vi "SSA_Template.vi"(0 "Reac Info":string[][](array[string])=[["Degradation_GFP", "", "false", "false", "Cell", "1", "GFP", "1.0", "true", "0", "", "", "0", "", "1", "kd", "0.0075"], ["Degradation_TetR", "", "false", "false", "Cell", "1", "TetR", "1.0", "true", "0", "", "", "0", "", "1", "kd", "0.0075"], ["Degradation_LacI", "", "false", "false", "Cell", "1", "LacI", "1.0", "true", "0", "", "", "0", "", "1", "kd", "0.0075"], ["R_abstracted_production_P1", "", "false", "false", "Cell", "0", "", "", "true", "1", "GFP", "10.0", "1", "LacI", "6", "RNAP, ng__P1, Ko__P1, ko__P1, nc__LacI_P1, Kr__LacI_P1", "30.0, 2.0, 0.033, 0.05, 2.0, 0.5"], ["R_abstracted_production_P2", "", "false", "false", "Cell", "0", "", "", "true", "1", "GFP", "10.0", "1", "TetR", "6", "RNAP, ng__P2, Ko__P2, ko__P2, nc__TetR_P2, Kr__TetR_P2", "30.0, 2.0, 0.033, 0.05, 2.0, 0.5"]], 1 "Ex_Mod_IDs":string[](array[string])=["LacI", "TetR"], 2 "Idx of Mod in Sp IDs":i32[](array[numeric])=[1, 4], 5 "Math Expressions":string[](array[string])=["kd*GFP", "kd*TetR", "kd*LacI", "ko__P1*ng__P1*Ko__P1*RNAP/(1+Ko__P1*RNAP+(Kr__LacI_P1*LacI)^nc__LacI_P1)", "ko__P2*ng__P2*Ko__P2*RNAP/(1+Ko__P2*RNAP+(Kr__TetR_P2*TetR)^nc__TetR_P2)"], 7 "Species Info":string[][](array[string])=[["GFP", "", "Cell", "0.0", "NaN", "", "true", "false", "false", "null"], ["LacI", "", "Cell", "0.0", "NaN", "", "true", "true", "false", "null"], ["P1", "", "Cell", "2.0", "NaN", "", "true", "false", "false", "null"], ["P2", "", "Cell", "2.0", "NaN", "", "true", "false", "false", "null"], ["TetR", "", "Cell", "0.0", "NaN", "", "true", "true", "false", "null"]], 9 "Parameter info":string[][](array[string])=[["ko_r", "Reverse RNAP binding rate", "1.0", "", "true"], ["nr", "Initial RNAP count", "30.0", "", "true"], ["np", "Stoichiometry of production", "10.0", "", "true"], ["kr_r", "Reverse repression binding rate", "1.0", "", "true"], ["ka_f", "Forward activation binding rate", "0.0033", "", "true"], ["kecdiff", "Extracellular diffusion rate", "1.0", "", "true"], ["ko", "Open complex production rate", "0.05", "", "true"], ["kmdiff_f", "Forward membrane diffusion rate", "1.0", "", "true"], ["kecd", "Extracellular degradation rate", "0.005", "", "true"], ["kc_r", "Reverse complex formation rate", "1.0", "", "true"], ["kr_f", "Forward repression binding rate", "0.5", "", "true"], ["ka_r", "Reverse activation binding rate", "1.0", "", "true"], ["nc", "Stoichiometry of binding", "2.0", "", "true"], ["kao_r", "Reverse activated RNAP binding rate", "1.0", "", "true"], ["kd", "Degradation rate", "0.0075", "", "true"], ["kb", "Basal production rate", "1.0E-4", "", "true"], ["ng", "Initial promoter count", "2.0", "", "true"], ["ka", "Activated production rate", "0.25", "", "true"], ["kao_f", "Forward activated RNAP binding rate", "1.0", "", "true"], ["kmdiff_r", "Reverse membrane diffusion rate", "0.01", "", "true"], ["ko_f", "Forward RNAP binding rate", "0.033", "", "true"], ["kc_f", "Forward complex formation rate", "0.05", "", "true"], ["High", "", "120.0", "", "true"], ["HighTime", "", "1000.0", "", "true"], ["HighTime2", "", "2000.0", "", "true"]], 11 "Local Parameter Info":string[][](array[string])=[["kd", "0.0075"], ["kd", "0.0075"], ["kd", "0.0075"], ["RNAP", "30.0"], ["ng__P1", "2.0"], ["Ko__P1", "0.033"], ["ko__P1", "0.05"], ["nc__LacI_P1", "2.0"], ["Kr__LacI_P1", "0.5"], ["RNAP", "30.0"], ["ng__P2", "2.0"], ["Ko__P2", "0.033"], ["ko__P2", "0.05"], ["nc__TetR_P2", "2.0"], ["Kr__TetR_P2", "0.5"]]) -> ()   [LabVIEW 2014]
uses:
  <vilib>/Analysis/Matrix/Datatypes/RealMatrix.ctl
  Modifier Control.ctl
  Event Info.ctl
  <vilib>/Utility/error.llb/DialogType.ctl
  ValSubsCtrl.ctl
  Trigger Status Bar.vi
  <vilib>/Utility/file.llb/Write To Spreadsheet File (DBL).vi
  <vilib>/Utility/file.llb/Write To Spreadsheet File (string).vi
  <vilib>/Analysis/Matrix/Numeric/Conversions/Matrix To Array - RM.vi
  <vilib>/regexp/Match Regular Expression.xnode
  <vilib>/Analysis/Matrix/NI_Matrix.lvlib
  <vilib>/gmath/NI_Gmath.lvlib
  <vilib>/Utility/file.llb/Read From Spreadsheet File (DBL).vi
panel:
  out "Reaction Math":string[][](array[string])
  out "Trig  MSW":bool=TRUE
  out "Plot colors":u32[](array[numeric])
  out "Plot Names":string[](array[string])
  out "Sp_Init_Amnt":string[](array[string])
  out "Trig Ext Mod Selection":bool=TRUE
  out "FuncCnt":i32
  out "Functions":string[][](array[string])
  out "Fn Arg Cnt":string[](array[string])
  out "Priority":dbl[](array[numeric])
  out "Delay Val Tot":dbl[](array[numeric])
  out "Flag":i32[](array[numeric])
  out "Delay":dbl[](array[numeric])
  out "Delay Val":dbl
  out "Event Idx":i32
  out "All Variables":string[](array[string])
  out "Time Limit":dbl
  out "ModTimeSym":string
  out "CompSize":string[](array[string])
  out "CompID":string[](array[string])
  out "Comp Def":string[][](array[string])
  out "Rules":string[][](array[string])
  out "RulesCnt":i32
  in  "Run":bool
  in  "stop":bool
  in  "Stop Main":bool
  out "Sp_Name":string[](array[string])
  out "Reac IDx":i32
  out "T=inf":bool
  out "Nxt Sp State (N)":dbl[](array[numeric])
  out "Propensities":dbl[](array[numeric])
  out "tau":dbl
  out "T":dbl[](array[numeric])
  out "Nxt T":dbl
  out "AppPath":string
  out "path":path
  in  "Shut Down":bool
  out "Default Stoich":dbl[](array[numeric])
  in  "Event Info":T1
  in  "Model Name 2":string="nand_RB"
  in  "Model Name":string="nand_RB"
  out "Reactant Matrix":T2
  out "Sp Ids":string[](array[string])
  out "Delta Matrix":T2
  out "XY Graph":cluster{"T":dbl[], dbl[]}[](graph)
  in  "Include Cello UCF":bool
  in  "Set Time Limit":string="100"
  in  "Continous Simulation":bool
  in  "Simulate SBML Events":bool
  in  "Threshold Value Analysis":bool
  in  "Modifier Degradation":bool
  in  "Slider":bool
  out "Assign Val":string[][](array[string])
  out "Var Idx":i32[](array[numeric])
  out "output array":T2
  out "RulVarIdx":i32[](array[numeric])
  out "DelMatRul":T2
  out "Init Sp State (S)":string[](array[string])
  out "DelMatOrigSize":i32
  out "Assign Var Idx":i32[][](array[numeric])
  out "Math Op":string[](array[string])
  out "Math Val":string[](array[string])
  in  "Events Info":string[][](table)=[["event0", "true", "true", "true", "t >= HighTime", "TetR = High"], ["event1", "true", "true", "true", "t >= HighTime2", "LacI = High"]]
  out "Log Data matrix":dbl[][](array[numeric]) format="%0.3f"
  out "All Param IDs":string[](array[string])
  out "All Param Vals":string[](array[string])
  out "Log Data":dbl[](array[numeric])
  out "Reac to execute":dbl[](array[numeric])
  out "Output Equations":string[](array[string])
  out "Nxt Sp State (S)":string[](array[string])
  out "All Param Names":string[](array[string])
  out "Equations":string[](array[string])
  out "Init Sp State (N)":dbl[](array[numeric])
  out "a0*r2":dbl
  out "Sum of Propensities for U":dbl
  out "Sum>a0*r2":bool
  out "r1":dbl
  out "L_cnt":i32
  out "r2":dbl
  out "a0":dbl
  out "Sp Data":dbl[][](array[numeric]) format="%0.3f"
  in  "External Modifiers":T3[](array[typedef]) {"Dial" scale=0.0..100.0 scale format="%#_3g"}
  in  "Boolean":bool=TRUE
  out "Est Thresh Val":dbl
  in  "Logic Verification":bool
  in  "Simulation Speed (ms)":u32=30
  out "DataLog":path
  out "All Param Values":string[](array[string])
  # "Virtual Laboratory Instrument for Stochastic Simulations"
  # "Settings"
  # "Yes"
  # "No"
  # "Manual"
  # "Auto"
  # "Model Parameters"
  # "Global Parameters"
  # "Local Parameters"
  # "ID"
  # "Name"
  # "Value"
  # "ID"
  # "Value"
  # "Runtime Simulation\nOptions"
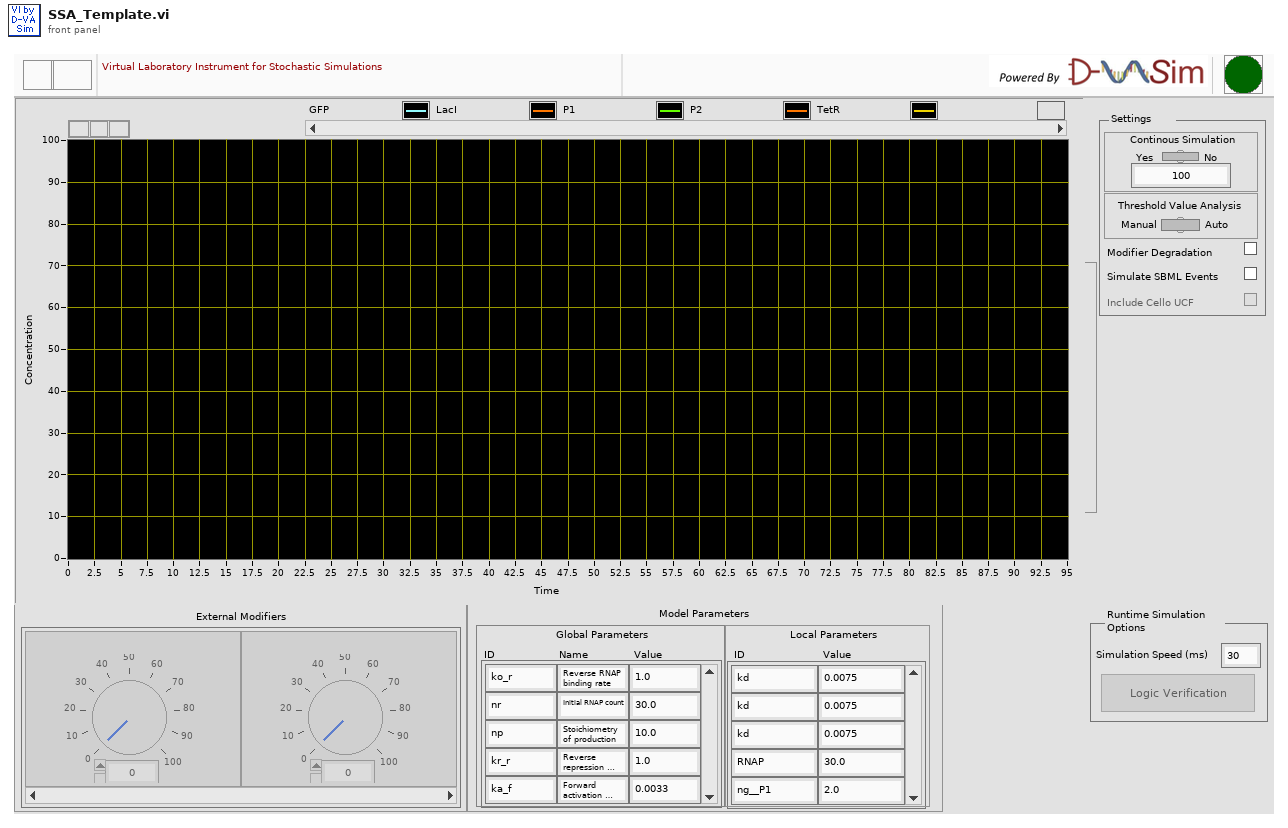
[diagram p1: front panel]
types:
  T1 = typedef "Event Info.ctl" = cluster{"Math Var":string[], "Math Op":string[], "Math Val":string[], "Assign Var":string[][], "Assign Op":string[][], "Assign Val":string[][], "Var Idx":i32[], "Assign Var Idx":i32[][], "Delay":string[], "Priority":string[]}
  T2 = typedef "NI_Matrix.lvlib/RealMatrix.ctl" = dbl[][]
  T3 = typedef "Modifier Control.ctl" = cluster{"Dial":dbl, "String 2":string}
  T4 = typedef "DialogType.ctl" = u16
  T5 = typedef "Model Information.ctl" = cluster{"ID":string, "Name":string, "Substance Units":string, "Time Units":string, "Volume Units":string, "Area Units":string, "Length Units":string, "Extent Units":string, "Conversion Factor":string, "Model Components":string}
  T6 = cluster{"Model Info":T5, "SpCnt":i32, "Species Info":string[][], "Pr_Cnt":i32, "Parameter info":string[][], "ReacCnt":i32, "Reaction Info":string[][], "Math Expressions":string[][], "EventsCnt":i32, "Event Info":string[][], "UnitsDefCnt":i32, "Units Def":string[][], "CompCnt":i32, "Comp Def":string[][], "Mod_ID":string[], "Mod_Idx":i32[], "RulesCnt":i32, "Rules":string[][], "FuncCnt":i32, "Functions":string[][], "InitAssign Cnt":i32, "Init Assigns":string[][], "ConstraintsCnt":i32, "Constraints":string[][], "Fn Arg Cnt":string[]}
  T7 = enum8{"Enabled", "Disabled", "Disabled and Grayed Out"}
  T8 = typedef "ValSubsCtrl.ctl" = cluster{"All Param Names":string[], "All Param Values":string[], "Sp IDs":string[], "Sp States":string[], "Input Equations":string[], "CompID":string[], "CompSize":string[], "T-Sym":string, "T":dbl}
  T9 = typedef "Threshold Set.ctl" = cluster{"Start at":dbl, "Increment of":dbl, "Stop at":dbl, "No. of iterations":dbl, "Assumed Time Delay":dbl, "Th high":dbl, "Verification RT":dbl, "Settling Time":i32, "Name of Output":string, "Th Low":dbl}
  T10 = enum32{"invalid app kind", "Development System", "Run Time System", "Student Edition", "Embedded LabVIEW", "Evaluation", "Custom"}
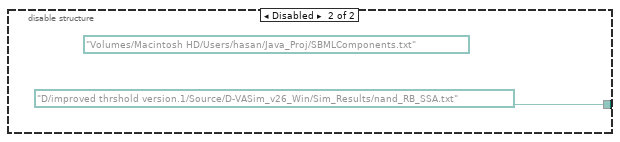
[diagram p2: hidden frame]
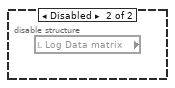
[diagram p3: hidden frame]
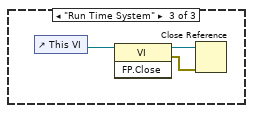
[diagram p5: hidden frame]
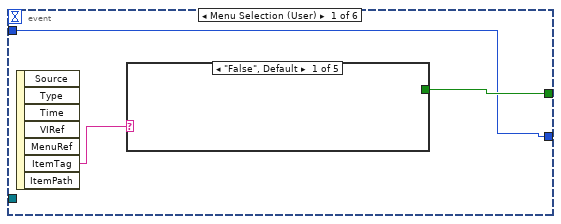
[diagram p6: hidden frame]
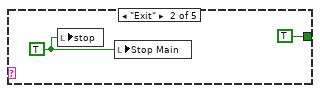
[diagram p7: hidden frame]
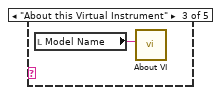
[diagram p8: hidden frame]
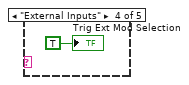
[diagram p9: hidden frame]
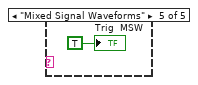
[diagram p10: hidden frame]
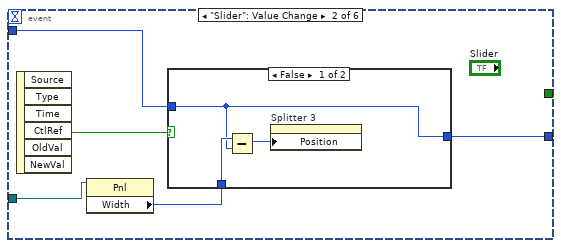
[diagram p11: hidden frame]
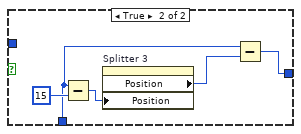
[diagram p12: hidden frame]
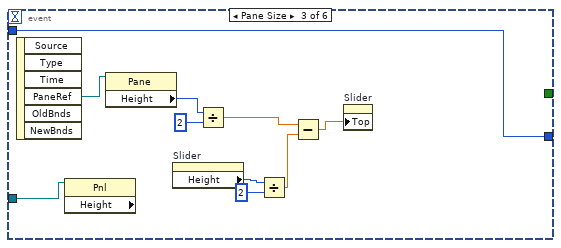
[diagram p13: hidden frame]
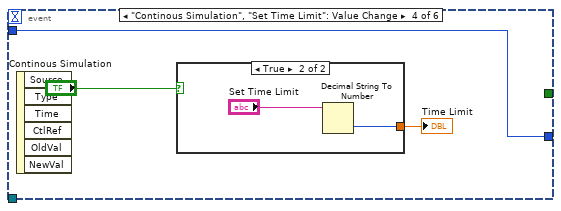
[diagram p14: hidden frame]
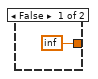
[diagram p15: hidden frame]
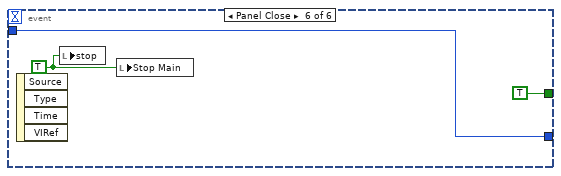
[diagram p16: hidden frame]
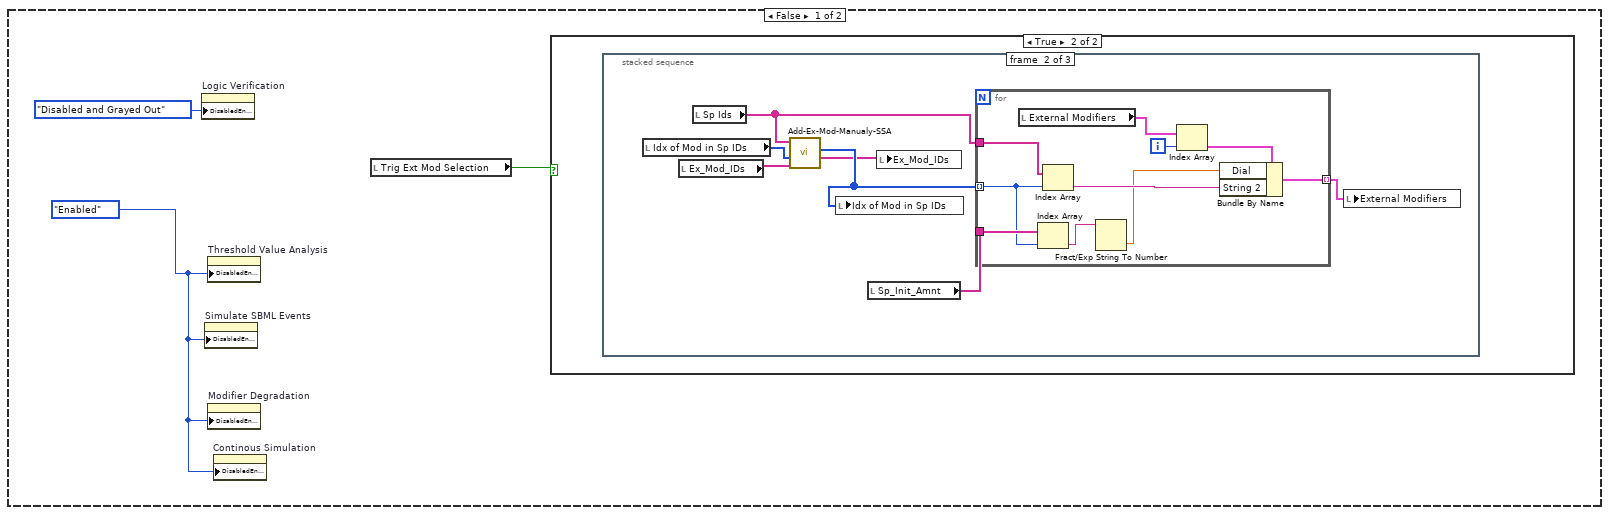
[diagram p17: hidden frame]
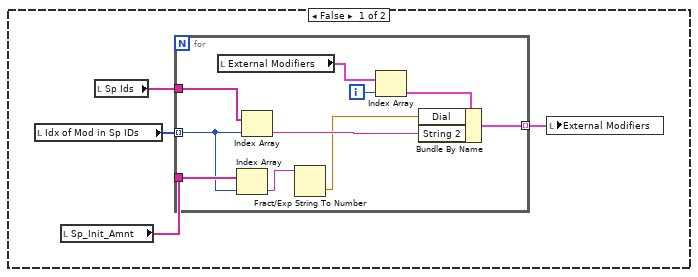
[diagram p18: hidden frame]
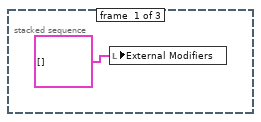
[diagram p19: hidden frame]
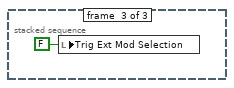
[diagram p20: hidden frame]
diagram:
  (unwired) 928 ("Splitter Position")
  w9 = T4 2 items=["no dialog", "OK message", "continue or stop message", "OK message + warnings", "continue/stop + warnings"] ("type of dialog (OK msg:1)")
  n1 = flat-sequence {
    tunnel: [w11] -> w4
    tunnel: w4 -> [w36]
    tunnel: [w69] -> w3
    frame #0 {
      n2 = Current VI's Path() -> (path=w21:path)
      n3 = Path To String(path=w21) -> (string=w20:string)
      n4 = Match Pattern(string=w20, regular expression="Sim_Results\\" ("string")) -> (before substring=w18:string)  [unwired: 1 in, 3 out]
      n5 = Concatenate Strings(w18, "Sim_Results\\" ("string")) -> (w16:string)
      "AppPath" <- w16
      n6 = disable-structure shown="Enabled" {
        disable-tunnel: [w31 path "D:/improved thrshold version.1/Source/D-VASim_v26_Win/Sim_Results/nand_RB_SSA.txt" ("SBML File")] -> w11
        disable-tunnel: w16 -> [w22 _]
        frame Enabled {
          # "Reference convert into path"
          n7 = control-ref of="This VI"() -> (w30:refnum<vi>)
          n8 = property class="VI"(reference=w30) -> ("Name"=w29:string)  [unwired: 1 in, 2 out]
          n9 = Search and Replace String(input string=w29, search string=".vi", replace string="") -> (result string=w26:string)  [unwired: 5 in, 3 out]
          n10 = Concatenate Strings(w26, ".txt" ("search string")) -> (w24:string)
          n11 = local write "Model Name"(w26) -> ()
          n12 = Concatenate Strings(w22, w24) -> (w23:string)
          n13 = String To Path(string=w23) -> (path=w31:path)
        }
        frame Disabled {
          (unwired) path "/Volumes/Macintosh HD/Users/hasan/Java_Proj/SBMLComponents.txt" ("SBML File")
        }
      }
      "path" <- w11
      n14 = property on="XY Graph" class="XYGraph (strict)"("LegScrollVis"=TRUE ("Legend:Scrollbar Visible")) -> ()  [unwired: 2 in, 2 out]
      n15 = property on="XY Graph" class="XYGraph (strict)"("LegAutosize"=FALSE ("Legend:Autosize"), "Plot.Plot Name"="") -> ()  [unwired: 2 in, 2 out]
      n16 = local write "Trig  MSW"(FALSE ("Trig  MSW")) -> ()
    }
    frame #1 {
      # "Switch to threshold analysis"
      # "here SBML.vi data get and display in front end."
      n17 = call "SBML_File_Parser.vi"("SBML File"=w36) -> ("SBML Data"=w64:T6)  [unwired: 17 in, 1 out]
      n18 = Unbundle By Name(w64) -> ("Model Info.Time Units"=w57:string, "Species Info"=w44:string[][], "Parameter info"=w45:string[][], "Reaction Info"=w46:string[][], "Math Expressions"=w34:string[][], "Event Info"=w49:string[][], "Mod_ID"=w50:string[], "Mod_Idx"=w51:i32[], "RulesCnt"=→"RulesCnt":i32, "Rules"=→"Rules":string[][], "Comp Def"=→"Comp Def":string[][])
      "Reaction Math" <- w34
      n19 = Unbundle By Name(w64) -> ("FuncCnt"=→"FuncCnt":i32, "Functions"=→"Functions":string[][], "Fn Arg Cnt"=→"Fn Arg Cnt":string[])
      n20 = local write "Continous Simulation"(FALSE ("Continous Simulation")) -> ()
      n21 = Equal?(x="", y=w57) -> (x = y?=w55:bool)
      n22 = local write "Time Limit"(inf) -> ()
      n23 = local write "Species Info"(w44) -> ()
      n24 = local write "Parameter info"(w45) -> ()
      n25 = Select(t="undefined", s=w55, f=w57) -> (s? t:f=→"ModTimeSym":string)
      n26 = local write "Reac Info"(w46) -> ()
      n27 = Index Array(array=w46, index (col)=17 ("disabled index (col)")) -> (element=w48:string[])  [unwired: 1 in]
      n28 = Index Array(array=w34, index (col)=1 ("disabled index (col)")) -> (element=w35:string[])  [unwired: 1 in]
      n29 = Index Array(array=w46, index (col)=16 ("disabled index (col)")) -> (element=w47:string[])  [unwired: 1 in]
      n30 = local write "Events Info"(w49) -> ()
      n31 = local write "Ex_Mod_IDs"(w50) -> ()
      n32 = local write "Idx of Mod in Sp IDs"(w51) -> ()
      n33 = call "Comma-separated-list extractor.vi"("In_list"=w47) -> ("List_Out"=w41:string[])  [unwired: 6 in, 1 out]
      n34 = call "Comma-separated-list extractor.vi"("In_list"=w48) -> ("List_Out"=w42:string[])  [unwired: 6 in, 1 out]
      n35 = Build Array(w41, w42) -> (w40:string[][])
      n36 = Transpose 2D Array(2D array=w40) -> (transposed array=w43:string[][])
      n37 = local write "Math Expressions"(w35) -> ()
      n38 = local write "Local Parameter Info"(w43) -> ()
    }
    frame #2 {
      # "run time value (Knob)"
      # "External Interfaces"
      n39 = local read "Species Info"() -> (w67:string[][])
      n40 = local read "Idx of Mod in Sp IDs"() -> (w72:i32[])
      n41 = Index Array(array=w67, index (col)=3 ("disabled index (col)")) -> (element=w66:string[])  [unwired: 1 in]
      "Sp_Init_Amnt" <- w66
      n42 = Index Array(array=w67, index (col)=0 ("disabled index (col)")) -> (element=w70:string[])  [unwired: 1 in]
      "Sp Ids" <- w70
      n43 = for {
        tunnel: w72 -> [w74] mode=indexing
        tunnel: w70 -> [w82]
        tunnel: [w77] -> w69 mode=indexing
        tunnel: w66 -> [w75]
        i -> [w80]
        n44 = local read "External Modifiers"() -> (w81:T3[])
        n45 = Index Array(array=w75, index=w74) -> (element=w76:string)
        n46 = Index Array(array=w82, index=w74) -> (element=w78:string)
        n47 = Fract/Exp String To Number(string=w76) -> (number=w73:dbl)  [unwired: 3 in, 1 out]
        n48 = Index Array(array=w81, index=w80) -> (element=w79:T3)
        n49 = Bundle By Name(cluster=w79, "Dial"=w73, "String 2"=w78) -> (w77:T3)
      }
      n50 = local write "Trig Ext Mod Selection"(FALSE ("Trig Ext Mod Selection")) -> ()
      n51 = local write "External Modifiers"(w69) -> ()
    }
  }
  n52 = while {
    tunnel: ["Stop Main"] -> w6
    tunnel: w3 -> [_]
    stop <- "Stop Main" stop-if-true
    # "start analysis (Start Button)"
    n53 = Wait Until Next ms Multiple(millisecond multiple=u32 50) -> ()  [unwired: 1 out]
    n54 = case shown="True" "Run" {
      frame False {
        w87 = T7."Enabled" ("Disabled")
        n55 = property on="Logic Verification" class="Bool (strict)"("DisabledEnum"=T7."Disabled and Grayed Out" ("Disabled")) -> ()  [unwired: 2 in, 2 out]
        n56 = property on="Simulate SBML Events" class="Bool (strict)"("DisabledEnum"=w87) -> ()  [unwired: 2 in, 2 out]
        n57 = property on="Threshold Value Analysis" class="Bool (strict)"("DisabledEnum"=w87) -> ()  [unwired: 2 in, 2 out]
        n58 = property on="Modifier Degradation" class="Bool (strict)"("DisabledEnum"=w87) -> ()  [unwired: 2 in, 2 out]
        n59 = property on="Continous Simulation" class="Bool (strict)"("DisabledEnum"=w87) -> ()  [unwired: 2 in, 2 out]
        n60 = local read "Trig Ext Mod Selection"() -> (w86:bool)
        n61 = case shown="True" w86 {
          frame False {
            n62 = local read "Idx of Mod in Sp IDs"() -> (w91:i32[])
            n63 = local read "Sp_Init_Amnt"() -> (w89:string[])
            n64 = local read "Sp Ids"() -> (w90:string[])
            n65 = for {
              tunnel: w91 -> [w94] mode=indexing
              tunnel: w90 -> [w102]
              tunnel: [w97] -> w92 mode=indexing
              tunnel: w89 -> [w95]
              i -> [w100]
              n66 = local read "External Modifiers"() -> (w101:T3[])
              n67 = Index Array(array=w95, index=w94) -> (element=w96:string)
              n68 = Index Array(array=w102, index=w94) -> (element=w98:string)
              n69 = Fract/Exp String To Number(string=w96) -> (number=w93:dbl)  [unwired: 3 in, 1 out]
              n70 = Index Array(array=w101, index=w100) -> (element=w99:T3)
              n71 = Bundle By Name(cluster=w99, "Dial"=w93, "String 2"=w98) -> (w97:T3)
            }
            n72 = local write "External Modifiers"(w92) -> ()
          }
          frame True {
            n73 = stacked-sequence {
              frame #0 {
                n74 = local write "External Modifiers"(T3[] [] ("Modifiers Array")) -> ()
              }
              frame #1 {
                n75 = local read "Idx of Mod in Sp IDs"() -> (w104:i32[])
                n76 = local read "Ex_Mod_IDs"() -> (w107:string[])
                n77 = local read "Sp Ids"() -> (w105:string[])
                n78 = call "Add-Ex-Mod-Manualy-SSA.vi"("In-Ex_Mod_IDs"=w107, "In-Idx of Mod in Sp IDs"=w104, "Sp IDs"=w105) -> ("Out-Ex_Mod_IDs"=w106:string[], "O/p Idx of Mod in Sp IDs"=w108:i32[])  [unwired: 7 in]
                n79 = local write "Idx of Mod in Sp IDs"(w108) -> ()
                n80 = local read "Sp_Init_Amnt"() -> (w109:string[])
                n81 = local write "Ex_Mod_IDs"(w106) -> ()
                n82 = for {
                  tunnel: w108 -> [w112] mode=indexing
                  tunnel: w105 -> [w120]
                  tunnel: [w115] -> w110 mode=indexing
                  tunnel: w109 -> [w113]
                  i -> [w118]
                  n83 = local read "External Modifiers"() -> (w119:T3[])
                  n84 = Index Array(array=w113, index=w112) -> (element=w114:string)
                  n85 = Index Array(array=w120, index=w112) -> (element=w116:string)
                  n86 = Fract/Exp String To Number(string=w114) -> (number=w111:dbl)  [unwired: 3 in, 1 out]
                  n87 = Index Array(array=w119, index=w118) -> (element=w117:T3)
                  n88 = Bundle By Name(cluster=w117, "Dial"=w111, "String 2"=w116) -> (w115:T3)
                }
                n89 = local write "External Modifiers"(w110) -> ()
              }
              frame #2 {
                n90 = local write "Trig Ext Mod Selection"(FALSE ("Trig Ext Mod Selection")) -> ()
              }
            }
          }
        }
      }
      frame True {
        (unwired) dbl[][] [] ("History Data")
        # "continous switch disable"
        n91 = local write "T=inf"(FALSE ("T=inf")) -> ()
        n92 = property on="Continous Simulation" class="Bool (strict)"("DisabledEnum"=T7."Disabled" ("Disabled")) -> ()  [unwired: 2 in, 2 out]
        n93 = invoke on="XY Graph" class="XYGraph (strict)" method="Reinit To Default"() -> ()  [unwired: 3 in, 3 out]
        n94 = stacked-sequence {
          seq-local: [_ _ _ w499 _ _ _ _ _ _] -> [_ _ _ _ _ _ _ _ _ w965]
          frame #0 {
            w149 = T7."Disabled" ("Disabled")
            w147 = T2 [] ("Reactant Matrix")
            w144 = string[] [] ("Init Sp State (S)")
            w146 = 0 ("Reac IDx")
            # "Internal controls"
            n95 = global write "Trigger Status Bar.vi" "Trigger Status Bar"(FALSE ("Trigger Status Bar 2")) -> ()
            n96 = property on="Logic Verification" class="Bool (strict)"("DisabledEnum"=T7."Enabled" ("Disabled")) -> ()  [unwired: 2 in, 2 out]
            n97 = local write "XY Graph"(cluster{"T":dbl[], dbl[]}[] [] ("XY Graph")) -> ()
            n98 = property on="Simulate SBML Events" class="Bool (strict)"("DisabledEnum"=w149) -> ()  [unwired: 2 in, 2 out]
            n99 = property on="Threshold Value Analysis" class="Bool (strict)"("DisabledEnum"=w149) -> ()  [unwired: 2 in, 2 out]
            n100 = property on="Modifier Degradation" class="Bool (strict)"("DisabledEnum"=w149) -> ()  [unwired: 2 in, 2 out]
            n101 = local read "Sp Ids"() -> (w142:string[])
            n102 = Array Size(array=w142) -> (size(s)=w141:i32)
            n103 = Initialize Array(0.0 ("element"), w141) -> (→"Default Stoich":dbl[])
            "Equations" <- w144
            "r2" <- 0.0 ("r2")
            "tau" <- 0.0 ("tau")
            "T" <- dbl[] [0.0] ("T")
            "L_cnt" <- 0 ("L_cnt")
            "Propensities" <- dbl[] [] ("Propensities")
            "a0" <- 0.0 ("a0")
            "r1" <- 0.0 ("r1")
            "a0*r2" <- 0.0 ("a0*r2")
            "Reac IDx" <- w146
            "Delta Matrix" <- w147
            "Sum>a0*r2" <- FALSE ("Sum>a0*r2")
            "Log Data" <- dbl[] [] ("Log Data")
            "Output Equations" <- string[] [] ("Output Equations")
            "Sp Data" <- dbl[][] [] ("Sp Data")
            "Reac to execute" <- dbl[] [] ("Reac to execute")
            "Sum of Propensities for U" <- 0.0 ("Sum of Propensities")
            "Nxt T" <- 0.0 ("Last T")
            "Nxt Sp State (S)" <- w144
            "Init Sp State (S)" <- w144
            "Reactant Matrix" <- w147
            "Sp_Name" <- w144
            "Log Data matrix" <- w147
            "All Param Names" <- w144
            "All Param Values" <- w144
            "DelMatRul" <- w147
            "DelMatOrigSize" <- w146
            "RulVarIdx" <- i32[] [] ("RulVarIdx")
            "All Variables" <- w144
          }
          frame #1 {
            # "This sequence is added to make the SSA template without scripting"
            n104 = local read "FuncCnt"() -> (w167:i32)
            n105 = case shown="1.." w167 {
              selector: w167 -> [_ w172]
              frame 0, Default {
              }
              frame 1.. {
                n106 = local read "Fn Arg Cnt"() -> (w170:string[])
                n107 = local read "Functions"() -> (w171:string[][])
                n108 = local read "Math Expressions"() -> (w168:string[])
                n109 = call "Func Processor for K-Laws-16032016.vi"("Math Expressions In"=w168, "Fn Arg Cnt"=w170, "Functions Definition"=w171, "Total Function Definitions"=w172) -> ("Math Expressions Out"=w169:string[])  [unwired: 7 in]
                n110 = local write "Math Expressions"(w169) -> ()
              }
            }
          }
          frame #2 {
            # "P_Stoich"
            # "Products"
            # "R-Stoich"
            # "Sp IDs"
            # "Reactants"
            n111 = local read "Reac Info"() -> (w173:string[][])
            n112 = local read "Sp Ids"() -> (w180:string[])
            n113 = Index Array(array=w173, index (col)=10 ("disabled index (col)")) -> (element=w179:string[])  [unwired: 1 in]
            n114 = Index Array(array=w173, index (col)=6 ("disabled index (col)")) -> (element=w183:string[])  [unwired: 1 in]
            n115 = Index Array(array=w173, index (col)=7 ("disabled index (col)")) -> (element=w184:string[])  [unwired: 1 in]
            n116 = Index Array(array=w173, index (col)=11 ("disabled index (col)")) -> (element=w187:string[])  [unwired: 1 in]
            n117 = local read "Model Name"() -> (w178:string)
            n118 = local read "AppPath"() -> (w174:string)
            n119 = Concatenate Strings(w174, w178, "_Delta Matrix.xls") -> (w176:string)
            n120 = String To Path(string=w176) -> (path=w175:path)
            n121 = disable-structure shown="Enabled" {
              disable-tunnel: w187 -> [w193 w288]
              disable-tunnel: w184 -> [w192 w292]
              disable-tunnel: w183 -> [w191 w291]
              disable-tunnel: w180 -> [w190 w289]
              disable-tunnel: w179 -> [w189 w290]
              disable-tunnel: w175 -> [w188 w287]
              frame Disabled {
                n122 = stacked-sequence {
                  tunnel: w191 -> [w197 _]
                  tunnel: w190 -> [w196 w240]
                  tunnel: w192 -> [w195 _]
                  tunnel: w193 -> [_ w239]
                  tunnel: w189 -> [_ w238]
                  tunnel: w188 -> [w194 w237]
                  frame #0 {
                    n123 = for {
                      tunnel: w197 -> [w200] mode=indexing
                      tunnel: w196 -> [w204]
                      tunnel: w195 -> [w203] mode=indexing
                      tunnel: w194 -> [w198]
                      i -> [w202]
                      # "Reactants"
                      # "R-Stoich"
                      # "Specie"
                      n124 = Not Equal?(x=w200, y="") -> (x != y?=w199:bool)
                      n125 = case shown="True" w199 {
                        tunnel: w200 -> [_ w209]
                        tunnel: w204 -> [_ w208]
                        tunnel: w203 -> [_ w207]
                        tunnel: w202 -> [_ w206]
                        tunnel: w198 -> [_ w205]
                        frame False {
                        }
                        frame True {
                          n126 = for {
                            tunnel: w209 -> [w225]
                            tunnel: w208 -> [w214] mode=indexing
                            tunnel: w207 -> [w223]
                            tunnel: w206 -> [w219]
                            tunnel: w205 -> [w216]
                            i -> [w218]
                            n127 = Equal?(x=w214, y=w225) -> (x = y?=w213:bool)
                            n128 = case shown="False" w210 {
                              tunnel: [w231 w236] -> w212
                              tunnel: w214 -> [w230 _]
                              tunnel: w213 -> [w229 w236]
                              frame False {
                                n129 = local read "Ex_Mod_IDs"() -> (w235:string[])
                                n130 = Search 1D Array(1D array=w235, element=w230) -> (index of element=w233:i32)  [unwired: 1 in]
                                n131 = Equal?(x=w233, y=-1.0) -> (x = y?=w234:bool)
                                n132 = And(x=w229, y=w234) -> (x .and. y?=w231:bool)
                              }
                              frame True {
                              }
                            }
                            n133 = Decimal String To Number(string=w223, default (0L)=0.0 ("t")) -> (number=w221:dbl)  [unwired: 1 in, 1 out]
                            n134 = Multiply(x=-1.0 ("t"), y=w221) -> (x*y=w220:dbl)
                            n135 = local read "Delta Matrix"() -> (w211:T2)
                            n136 = Select(t=w220, s=w212, f=0.0 ("t")) -> (s? t:f=w217:dbl)
                            n137 = Replace Array Subset(array=w211, new element=w217, index (row)=w219, index (col)=w218) -> (w215:T2)
                            n138 = disable-structure shown="Enabled" {
                              disable-tunnel: w216 -> [w228 _]
                              disable-tunnel: w215 -> [w227 _]
                              frame Enabled {
                                n139 = call-poly <vilib>:"Write To Spreadsheet File.vi"("2D data"=w227, "file path (dialog if empty)"=w228) -> ()  [unwired: 6 in, 1 out]
                              }
                              frame Disabled {
                              }
                            }
                            n140 = local write "Delta Matrix"(w215) -> ()
                          }
                        }
                      }
                    }
                  }
                  frame #1 {
                    n141 = for {
                      tunnel: w238 -> [w243] mode=indexing
                      tunnel: w240 -> [w247]
                      tunnel: w239 -> [w246] mode=indexing
                      tunnel: w237 -> [w241]
                      i -> [w245]
                      # "P_Stoich"
                      # "Sp IDs"
                      # "Products"
                      n142 = Not Equal?(x=w243, y="") -> (x != y?=w242:bool)
                      n143 = case shown="True" w242 {
                        tunnel: w243 -> [_ w252]
                        tunnel: w247 -> [_ w251]
                        tunnel: w246 -> [_ w250]
                        tunnel: w245 -> [_ w249]
                        tunnel: w241 -> [_ w248]
                        frame False {
                        }
                        frame True {
                          n144 = for {
                            tunnel: w252 -> [w259]
                            tunnel: w251 -> [w260] mode=indexing
                            tunnel: w250 -> [w258]
                            tunnel: w249 -> [w257]
                            tunnel: w249 -> [w255]
                            tunnel: w248 -> [w253]
                            i -> [w254]
                            n145 = flat-sequence {
                              tunnel: w260 -> [w271]
                              tunnel: w259 -> [w270]
                              tunnel: w258 -> [w268]
                              tunnel: w257 -> [w263]
                              tunnel: w254 -> [w262]
                              tunnel: [w264] -> w256
                              tunnel: w256 -> [w280]
                              tunnel: w255 -> [w282]
                              tunnel: w254 -> [w281]
                              tunnel: w253 -> [w278]
                              frame #0 {
                                n146 = disable-structure shown="Enabled" {
                                disable-tunnel: w263 -> [w275 _]
                                disable-tunnel: w262 -> [w274 _]
                                disable-tunnel: [w273 0.0 ("Real Matrix Element")] -> w261
                                frame Disabled {
                                n147 = local read "Delta Matrix"() -> (w276:T2)
                                n148 = Index Array(array=w276, index (row)=w275, index (col)=w274) -> (element=w273:dbl)
                                }
                                frame Enabled {
                                }
                                }
                                n149 = Decimal String To Number(string=w268, default (0L)=0.0 ("t")) -> (number=w266:dbl)  [unwired: 1 in, 1 out]
                                n150 = Multiply(x=1.0 ("t"), y=w266) -> (x*y=w265:dbl)
                                n151 = Equal?(x=w271, y=w270) -> (x = y?=w272:bool)
                                n152 = Select(t=w265, s=w272, f=w261) -> (s? t:f=w264:dbl)
                              }
                              frame #1 {
                                n153 = local read "Delta Matrix"() -> (w283:T2)
                                n154 = Replace Array Subset(array=w283, new element=w280, index (row)=w282, index (col)=w281) -> (w279:T2)
                                n155 = disable-structure shown="Enabled" {
                                disable-tunnel: w279 -> [w285 _]
                                disable-tunnel: w278 -> [w284 _]
                                frame Enabled {
                                n156 = call-poly <vilib>:"Write To Spreadsheet File.vi"("2D data"=w285, "file path (dialog if empty)"=w284) -> ()  [unwired: 6 in, 1 out]
                                }
                                frame Disabled {
                                }
                                }
                                n157 = local write "Delta Matrix"(w279) -> ()
                              }
                            }
                          }
                        }
                      }
                    }
                  }
                }
              }
              frame Enabled {
                # "This code is modified on march 30 2016"
                n158 = for {
                  tunnel: w291 -> [w302] mode=indexing
                  tunnel: w289 -> [w306]
                  tunnel: w292 -> [w305] mode=indexing
                  tunnel: w290 -> [w296] mode=indexing
                  tunnel: w288 -> [w297] mode=indexing
                  tunnel: [w295] -> w286
                  i -> [w304]
                  # "P-stoich"
                  # "Products"
                  # "Reactants"
                  # "R-Stoich"
                  # "Specie"
                  # "Extracting the list of reactants and products of all reactions"
                  n159 = Not Equal?(x=w296, y="") -> (x != y?=w300:bool)
                  n160 = Not Equal?(x=w302, y="") -> (x != y?=w299:bool)
                  n161 = Or(x=w299, y=w300) -> (x .or. y?=w298:bool)
                  n162 = case shown="True" w298 {
                    tunnel: w302 -> [_ w313]
                    tunnel: w306 -> [_ w312]
                    tunnel: w305 -> [_ w311]
                    tunnel: w304 -> [_ w310]
                    tunnel: w297 -> [_ w309]
                    tunnel: w296 -> [_ w308]
                    tunnel: [_ w307] -> w295
                    frame False {
                    }
                    frame True {
                      n163 = stacked-sequence {
                        tunnel: w313 -> [w317 _ _]
                        tunnel: w311 -> [w320 _ _]
                        tunnel: w310 -> [w322 _ w408]
                        tunnel: w312 -> [w321 _ w409]
                        tunnel: w309 -> [_ _ w403]
                        tunnel: w308 -> [_ _ w406]
                        tunnel: [_ _ w407] -> w307
                        frame #0 {
                          n164 = Build Array(w320) -> (w319:string[])
                          n165 = Build Array(w317) -> (w316:string[])
                          n166 = call "Comma-separated-list extractor.vi"("In_list"=w319) -> ("List_Out"=w318:string[])  [unwired: 6 in, 1 out]
                          n167 = call "Comma-separated-list extractor.vi"("In_list"=w316) -> ("List_Out"=w315:string[])  [unwired: 6 in, 1 out]
                          n168 = Array Size(array=w315) -> (size(s)=w314:i32)
                          n169 = case shown="0, Default" w314 {
                            tunnel: w322 -> [w326 w365]
                            tunnel: w321 -> [w325 w364]
                            tunnel: w318 -> [w324 w363]
                            tunnel: w315 -> [w323 w362]
                            frame 1.. {
                              n170 = for {
                                tunnel: w326 -> [w330]
                                tunnel: w325 -> [w329]
                                tunnel: w324 -> [w328] mode=indexing
                                tunnel: w323 -> [w327] mode=indexing
                                # "Looping through all reactants of a current reaction"
                                n171 = for {
                                tunnel: w327 -> [w348]
                                tunnel: w328 -> [w346]
                                tunnel: w330 -> [w342]
                                tunnel: w329 -> [w340] mode=indexing
                                i -> [w333]
                                # "Looping through all species names"
                                n172 = Equal?(x=w340, y=w348) -> (x = y?=w339:bool)
                                n173 = case shown="False" "Modifier Degradation" {
                                tunnel: [w355 w360] -> w334
                                tunnel: w340 -> [w354 _]
                                tunnel: w339 -> [w353 w360]
                                tunnel: [w353 w360] -> w331
                                frame False {
                                n174 = local read "Ex_Mod_IDs"() -> (w359:string[])
                                n175 = Search 1D Array(1D array=w359, element=w354) -> (index of element=w357:i32)  [unwired: 1 in]
                                n176 = Equal?(x=w357, y=-1.0) -> (x = y?=w358:bool)
                                n177 = And(x=w353, y=w358) -> (x .and. y?=w355:bool)
                                }
                                frame True {
                                }
                                }
                                n178 = local read "Default Stoich"() -> (w336:dbl[])
                                n179 = Decimal String To Number(string=w346, default (0L)=0.0 ("t")) -> (number=w344:dbl)  [unwired: 1 in, 1 out]
                                n180 = Multiply(x=-1.0 ("t"), y=w344) -> (x*y=w343:dbl)
                                n181 = Index Array(array=w336, index=w333) -> (element=w335:dbl)
                                n182 = local read "Delta Matrix"() -> (w338:T2)
                                n183 = Select(t=w343, s=w334, f=w335) -> (s? t:f=w332:dbl)
                                n184 = Replace Array Subset(array=w338, new element=w332, index (row)=w342, index (col)=w333) -> (w341:T2)
                                n185 = local write "Delta Matrix"(w341) -> ()
                                n186 = case shown="True" w331 {
                                tunnel: w333 -> [_ w350]
                                tunnel: w332 -> [_ w349]
                                frame False {
                                }
                                frame True {
                                n187 = local read "Default Stoich"() -> (w351:dbl[])
                                n188 = Replace Array Subset(array=w351, new element=w349, index=w350) -> (w352:dbl[])
                                n189 = local write "Default Stoich"(w352) -> ()
                                }
                                }
                                }
                              }
                            }
                            frame 0, Default {
                              n190 = for {
                                N: 1 -> [_]
                                tunnel: w365 -> [w371]
                                tunnel: w364 -> [w370]
                                tunnel: w363 -> [w369]
                                tunnel: w362 -> [w367]
                                # "Looping through all reactants of a current reaction"
                                n191 = Index Array(array=w369) -> (element=w368:string)  [unwired: 1 in]
                                n192 = Index Array(array=w367) -> (element=w366:string)  [unwired: 1 in]
                                n193 = for {
                                tunnel: w366 -> [w386]
                                tunnel: w368 -> [w384]
                                tunnel: w371 -> [w380]
                                tunnel: w370 -> [w377] mode=indexing
                                i -> [w373]
                                # "Looping through all species names"
                                n194 = Equal?(x=w377, y=w386) -> (x = y?=w376:bool)
                                n195 = local read "Modifier Degradation"() -> (w372:bool)
                                n196 = case shown="False" w372 {
                                tunnel: [w390 w395] -> w375
                                tunnel: w377 -> [w389 _]
                                tunnel: w376 -> [w388 w395]
                                frame False {
                                n197 = local read "Ex_Mod_IDs"() -> (w394:string[])
                                n198 = Search 1D Array(1D array=w394, element=w389) -> (index of element=w392:i32)  [unwired: 1 in]
                                n199 = Equal?(x=w392, y=-1.0) -> (x = y?=w393:bool)
                                n200 = And(x=w388, y=w393) -> (x .and. y?=w390:bool)
                                }
                                frame True {
                                }
                                }
                                n201 = Decimal String To Number(string=w384, default (0L)=0.0 ("t")) -> (number=w382:dbl)  [unwired: 1 in, 1 out]
                                n202 = Multiply(x=-1.0 ("t"), y=w382) -> (x*y=w381:dbl)
                                n203 = local read "Delta Matrix"() -> (w374:T2)
                                n204 = Select(t=w381, s=w375, f=0.0 ("t")) -> (s? t:f=w379:dbl)
                                n205 = Replace Array Subset(array=w374, new element=w379, index (row)=w380, index (col)=w373) -> (w378:T2)
                                n206 = local write "Delta Matrix"(w378) -> ()
                                }
                              }
                            }
                          }
                        }
                        frame #1 {
                          n207 = local read "Sp Ids"() -> (w398:string[])
                          n208 = Array Size(array=w398) -> (size(s)=w397:i32)
                          n209 = Initialize Array(0.0 ("element"), w397) -> (w396:dbl[])
                          n210 = local write "Default Stoich"(w396) -> ()
                        }
                        frame #2 {
                          n211 = Build Array(w406) -> (w405:string[])
                          n212 = Build Array(w403) -> (w404:string[])
                          n213 = call "Comma-separated-list extractor.vi"("In_list"=w404) -> ("List_Out"=w402:string[])  [unwired: 6 in, 1 out]
                          n214 = call "Comma-separated-list extractor.vi"("In_list"=w405) -> ("List_Out"=w400:string[])  [unwired: 6 in, 1 out]
                          n215 = Array Size(array=w400) -> (size(s)=w401:i32)
                          n216 = case shown="0, Default" w401 {
                            tunnel: w409 -> [w414 w454]
                            tunnel: w408 -> [w413 w453]
                            tunnel: [w412 w452] -> w407
                            tunnel: w400 -> [w411 w451]
                            tunnel: w402 -> [w410 w450]
                            frame 1.. {
                              n217 = for {
                                tunnel: w410 -> [w419] mode=indexing
                                tunnel: w414 -> [w418]
                                tunnel: w411 -> [w417] mode=indexing
                                tunnel: w413 -> [w416]
                                tunnel: [w415] -> w412
                                # "Looping through all products of a current reaction"
                                n218 = for {
                                tunnel: w419 -> [w425]
                                tunnel: w418 -> [w424] mode=indexing
                                tunnel: w417 -> [w423]
                                tunnel: w416 -> [w422]
                                tunnel: [w421] -> w415
                                i -> [w420]
                                # "Looping through all species names"
                                n219 = flat-sequence {
                                tunnel: w424 -> [w437]
                                tunnel: w423 -> [w436]
                                tunnel: w425 -> [w434]
                                tunnel: [w430] -> w426
                                tunnel: w422 -> [w428]
                                tunnel: w420 -> [w427]
                                tunnel: w426 -> [w446]
                                tunnel: w422 -> [w447]
                                tunnel: w420 -> [w445]
                                tunnel: [w444] -> w421
                                frame #0 {
                                n220 = disable-structure shown="Enabled" {
                                disable-tunnel: w428 -> [w441 _]
                                disable-tunnel: w427 -> [w440 _]
                                disable-tunnel: [w439 0.0 ("Real Matrix Element")] -> w429
                                frame Enabled {
                                n221 = local read "Delta Matrix"() -> (w442:T2)
                                n222 = Index Array(array=w442, index (row)=w441, index (col)=w440) -> (element=w439:dbl)
                                }
                                frame Disabled {
                                }
                                }
                                n223 = Decimal String To Number(string=w434, default (0L)=0.0 ("t")) -> (number=w432:dbl)  [unwired: 1 in, 1 out]
                                n224 = Multiply(x=1.0 ("t"), y=w432) -> (x*y=w431:dbl)
                                n225 = Equal?(x=w437, y=w436) -> (x = y?=w438:bool)
                                n226 = Select(t=w431, s=w438, f=w429) -> (s? t:f=w430:dbl)
                                }
                                frame #1 {
                                n227 = local read "Delta Matrix"() -> (w448:T2)
                                n228 = Replace Array Subset(array=w448, new element=w446, index (row)=w447, index (col)=w445) -> (w444:T2)
                                n229 = local write "Delta Matrix"(w444) -> ()
                                }
                                }
                                }
                              }
                            }
                            frame 0, Default {
                              n230 = for {
                                N: 1 -> [_]
                                tunnel: w450 -> [w456]
                                tunnel: w454 -> [w459]
                                tunnel: w451 -> [w458]
                                tunnel: w453 -> [w461]
                                tunnel: [w460] -> w452
                                # "Looping through all products of a current reaction"
                                n231 = Index Array(array=w458) -> (element=w457:string)  [unwired: 1 in]
                                n232 = Index Array(array=w456) -> (element=w455:string)  [unwired: 1 in]
                                n233 = for {
                                tunnel: w455 -> [w467]
                                tunnel: w459 -> [w466] mode=indexing
                                tunnel: w457 -> [w465]
                                tunnel: w461 -> [w464]
                                tunnel: [w463] -> w460
                                i -> [w462]
                                # "Looping through all species names"
                                n234 = flat-sequence {
                                tunnel: w466 -> [w479]
                                tunnel: w465 -> [w478]
                                tunnel: w467 -> [w476]
                                tunnel: [w472] -> w468
                                tunnel: w464 -> [w470]
                                tunnel: w462 -> [w469]
                                tunnel: w468 -> [w488]
                                tunnel: w464 -> [w489]
                                tunnel: w462 -> [w487]
                                tunnel: [w486] -> w463
                                frame #0 {
                                n235 = disable-structure shown="Enabled" {
                                disable-tunnel: w470 -> [w483 _]
                                disable-tunnel: w469 -> [w482 _]
                                disable-tunnel: [w481 0.0 ("Real Matrix Element")] -> w471
                                frame Enabled {
                                n236 = local read "Delta Matrix"() -> (w484:T2)
                                n237 = Index Array(array=w484, index (row)=w483, index (col)=w482) -> (element=w481:dbl)
                                }
                                frame Disabled {
                                }
                                }
                                n238 = Decimal String To Number(string=w476, default (0L)=0.0 ("t")) -> (number=w474:dbl)  [unwired: 1 in, 1 out]
                                n239 = Multiply(x=1.0 ("t"), y=w474) -> (x*y=w473:dbl)
                                n240 = Equal?(x=w479, y=w478) -> (x = y?=w480:bool)
                                n241 = Select(t=w473, s=w480, f=w471) -> (s? t:f=w472:dbl)
                                }
                                frame #1 {
                                n242 = local read "Delta Matrix"() -> (w490:T2)
                                n243 = Replace Array Subset(array=w490, new element=w488, index (row)=w489, index (col)=w487) -> (w486:T2)
                                n244 = local write "Delta Matrix"(w486) -> ()
                                }
                                }
                                }
                              }
                            }
                          }
                        }
                      }
                    }
                  }
                }
                n245 = disable-structure shown="Enabled" {
                  disable-tunnel: w287 -> [w294 _]
                  disable-tunnel: w286 -> [w293 _]
                  frame Enabled {
                    n246 = call-poly <vilib>:"Write To Spreadsheet File.vi"("2D data"=w293, "file path (dialog if empty)"=w294) -> ()  [unwired: 6 in, 1 out]
                  }
                  frame Disabled {
                  }
                }
              }
            }
          }
          frame #3 {
            n247 = disable-structure shown="Disabled" {
              disable-tunnel: [w536 w542] -> w498
              frame Disabled {
                n248 = call <vilib>:"Application Directory.vi"() -> ("Application Directory"=w538:path)
                n249 = Path To String(path=w538) -> (string=w539:string)
                n250 = Concatenate Strings(w539, ":Sim_Results:", "Model Name") -> (w540:string)
                n251 = String To Path(string=w540) -> (path=w536:path)
              }
              frame Enabled {
                w546 = "DataLog.xls"
                n252 = local read "Model Name"() -> (w547:string)
                n253 = local read "AppPath"() -> (w548:string)
                n254 = Concatenate Strings(w548, w547, w546) -> (w550:string)
                n255 = String To Path(string=w550) -> (path=w543:path)
                n256 = String To Path(string=w548) -> (path=w549:path)
                n257 = List Folder(path=w549) -> (filenames=w545:string[])  [unwired: 3 in, 3 out]
                n258 = Concatenate Strings(w547, w546) -> (w544:string)
                n259 = for {
                  tunnel: w545 -> [w555] mode=indexing
                  tunnel: w544 -> [w554]
                  tunnel: w543 -> [w553]
                  tunnel: [w552] -> w542
                  stop <- w551 stop-if-true
                  n260 = Equal?(x=w555, y=w554) -> (x = y?=w556:bool)
                  n261 = case shown="True" w556 {
                    selector: w556 -> [w557 w559]
                    tunnel: w553 -> [w558 w561]
                    tunnel: [w558 w560] -> w552
                    tunnel: [w557 w559] -> w551
                    frame False {
                    }
                    frame True {
                      n262 = Delete(path (use dialog)=w561) -> (deleted path=w560:path)  [unwired: 4 in, 2 out]
                    }
                  }
                }
              }
            }
            n263 = disable-structure shown="Disabled" {
              disable-tunnel: [w530 _] -> _
              frame Disabled {
                n264 = call <vilib>:"Application Directory.vi"() -> ("Application Directory"=w528:path)
                n265 = call <vilib>:"Application Directory.vi"() -> ("Application Directory"=w532:path)
                n266 = Path To String(path=w528) -> (string=w529:string)
                n267 = Path To String(path=w532) -> (string=w533:string)
                n268 = Concatenate Strings(w529, ":Sim_Results:") -> (w526:string)
                n269 = Concatenate Strings(w533, ":Sim_Results:", "Model Name 2") -> (w534:string)
                n270 = String To Path(string=w526) -> ()  [unwired: 1 out]
                n271 = String To Path(string=w534) -> (path=w530:path)
              }
              frame Enabled {
              }
            }
            n272 = local read "Sp Ids"() -> (w505:string[])
            n273 = local read "AppPath"() -> (w497:string)
            n274 = flat-sequence {
              tunnel: w505 -> [w518]
              tunnel: [w518] -> w495
              tunnel: w495 -> [w519]
              frame #0 {
                n275 = Array Size(array=w518) -> (size(s)=w516:i32)
                n276 = property on="XY Graph" class="XYGraph (strict)"("LegAutosize"=FALSE ("Legend:Autosize"), "LegPlotMin"=w516) -> ()  [unwired: 2 in, 2 out]
              }
              frame #1 {
                n277 = for {
                  tunnel: w519 -> [w522] mode=indexing
                  tunnel: [w523] -> w521 mode=indexing
                  tunnel: [w522] -> w520 mode=indexing
                  i -> [w524]
                  n278 = property on="XY Graph" class="XYGraph (strict)"("Active Plot"=w524, "Plot.Line Width"=u8 2, "Plot.Plot Name"=w522) -> ("Plot.Plot Color"=w523:u32)  [unwired: 2 in, 2 out]
                }
                "Plot Names" <- w520
                "Plot colors" <- w521
              }
            }
            n279 = String To Path(string=w497) -> (path=w496:path)
            n280 = Insert Into Array(array=w505, index=0, new element="Time" ("string")) -> (w506:string[])
            n281 = local read "Model Name"() -> (w503:string)
            n282 = call-poly <vilib>:"Write To Spreadsheet File.vi"("1D data"=w506, "file path (dialog if empty)"=w498) -> ("new file path (Not A Path if cancelled)"=→"DataLog":path)  [unwired: 6 in]
            n283 = local read "Reaction Math"() -> (w494:string[][])
            n284 = Concatenate Strings(w503, "_" ("string"), "Screenshot" ("name or relative path")) -> (w500:string)
            n285 = Build Path(base path=w496, name or relative path=w500) -> (appended path=w499:path)
            n286 = case shown="True" "Include Cello UCF" {
              tunnel: w494 -> [w510 w515]
              tunnel: [w510 w512] -> w493
              tunnel: [w509 w513] -> w492
              frame False {
                n287 = Index Array(array=w510, index (col)=1 ("disabled index (col)")) -> (element=w509:string[])  [unwired: 1 in]
              }
              frame True {
                n288 = call "BU-Process-KLaws.vi"("Original Set of equations"=w515) -> ("Output Equations w param"=w512:string[][])  [unwired: 9 in, 1 out]
                n289 = Index Array(array=w512, index (col)=1 ("disabled index (col)")) -> (element=w513:string[])  [unwired: 1 in]
              }
            }
            n290 = local write "Math Expressions"(w492) -> ()
            n291 = local write "Reaction Math"(w493) -> ()
          }
          frame #4 {
            n292 = local read "Species Info"() -> (w585:string[][])
            n293 = local read "Math Expressions"() -> (w584:string[])
            n294 = Index Array(array=w585, index (col)=3 ("disabled index (col)")) -> (element=w563:string[])  [unwired: 1 in]
            n295 = local write "Equations"(w584) -> ()
            n296 = Array Size(array=w563) -> (size(s)=w565:i32)
            n297 = local read "Local Parameter Info"() -> (w569:string[][])
            n298 = Initialize Array("NaN" ("List of Reactions"), w565) -> (w564:string[])
            n299 = local read "Comp Def"() -> (w581:string[][])
            n300 = local read "Parameter info"() -> (w570:string[][])
            n301 = Equal?(x=w563, y=w564) -> (x = y?=w562:bool)
            n302 = Index Array(array=w581, index (col)=0 ("disabled index (col)")) -> (element=→"CompID":string[])  [unwired: 1 in]
            n303 = Index Array(array=w581, index (col)=3 ("disabled index (col)")) -> (element=→"CompSize":string[])  [unwired: 1 in]
            n304 = case shown="False" w562 {
              tunnel: w563 -> [_ w592]
              frame True {
                n305 = local read "Species Info"() -> (w589:string[][])
                n306 = Index Array(array=w589, index (col)=4 ("disabled index (col)")) -> (element=w587:string[])  [unwired: 1 in]
                n307 = Fract/Exp String To Number(string=w587) -> (number=w591:dbl[])  [unwired: 3 in, 1 out]
                n308 = local write "Init Sp State (S)"(w587) -> ()
                n309 = local write "Init Sp State (N)"(w591) -> ()
                n310 = local write "Nxt Sp State (N)"(w591) -> ()
                n311 = Number To Fractional String(number=w591) -> (F-format string=w590:string[])  [unwired: 3 in]
                n312 = local write "Nxt Sp State (S)"(w590) -> ()
              }
              frame False {
                n313 = Fract/Exp String To Number(string=w592) -> (number=w594:dbl[])  [unwired: 3 in, 1 out]
                n314 = local write "Init Sp State (S)"(w592) -> ()
                n315 = local write "Init Sp State (N)"(w594) -> ()
                n316 = local write "Nxt Sp State (N)"(w594) -> ()
                n317 = Number To Fractional String(number=w594) -> (F-format string=w593:string[])  [unwired: 3 in]
                n318 = local write "Nxt Sp State (S)"(w593) -> ()
              }
            }
            n319 = Index Array(array=w570, index (col)=0 ("disabled index (col)")) -> (element=w576:string[])  [unwired: 1 in]
            n320 = Index Array(array=w569, index (col)=0 ("disabled index (col)")) -> (element=w575:string[])  [unwired: 1 in]
            n321 = Index Array(array=w570, index (col)=2 ("disabled index (col)")) -> (element=w573:string[])  [unwired: 1 in]
            n322 = Index Array(array=w569, index (col)=1 ("disabled index (col)")) -> (element=w574:string[])  [unwired: 1 in]
            n323 = Build Array (concatenate)(w576, w575) -> (→"All Param IDs":string[])
            n324 = Build Array (concatenate)(w573, w574) -> (→"All Param Vals":string[])
          }
          frame #5 {
            # "Checking if Rules are present. If they are present, then insert rules into their respective species index."
            n325 = local read "RulesCnt"() -> (w602:i32)
            n326 = Not Equal?(x=w602, y=0) -> (x != y?=w600:bool)
            n327 = case shown="False" w600 {
              tunnel: [_ w605] -> w598
              frame False {
              }
              frame True {
                n328 = local read "Rules"() -> (w608:string[][])
                n329 = for {
                  tunnel: w608 -> [w613] mode=indexing
                  tunnel: [w611] -> w605
                  tunnel: [w610] -> w603 mode=indexing
                  i -> [w612]
                  n330 = Index Array(array=w613, index=0 ("disabled index (col)")) -> (element=w618:string)
                  n331 = Equal?(x=w618, y="rateRule") -> (x = y?=w615:bool)
                  n332 = Equal?(x=w618, y="assignmentRule") -> (x = y?=w616:bool)
                  n333 = Or(x=w615, y=w616) -> (x .or. y?=w614:bool)
                  n334 = case shown="True" w614 {
                    tunnel: w613 -> [_ w628]
                    tunnel: w612 -> [_ w625]
                    tunnel: [_ w623] -> w611
                    tunnel: [_ w622] -> w610
                    frame False {
                    }
                    frame True {
                      # "Extracting Rule"
                      # "Extracting Sp ID"
                      # "Inserting the rule in equations array"
                      # "Searching the index of Sp \nin Sp ID array"
                      # "If the rules is explicit (i.e. either rate or assignment rule) then extract the name of variable, then its index in the list of species and then put the rule math at that index in the equations array"
                      n335 = Index Array(array=w628, index=2 ("disabled index (col)")) -> (element=w632:string)
                      n336 = Index Array(array=w628, index=3 ("disabled index (col)")) -> (element=w627:string)
                      n337 = local read "Sp Ids"() -> (w633:string[])
                      n338 = Search 1D Array(1D array=w633, element=w632) -> (index of element=w622:i32)  [unwired: 1 in]
                      n339 = local read "Equations"() -> (w631:string[])
                      n340 = local read "DelMatRul"() -> (w626:T2)
                      n341 = Insert Into Array(array=w631, index=0, new element=w627) -> (w630:string[])
                      n342 = local write "Equations"(w630) -> ()
                      n343 = Replace Array Subset(array=w626, new element=1.0 ("element"), index (row)=w625, index (col)=w622) -> (w623:T2)
                      n344 = local write "DelMatRul"(w623) -> ()
                    }
                  }
                }
                n345 = Matrix Size(0:w608) -> (1:w604:i32, 2:w607:i32)
                n346 = local write "DelMatOrigSize"(w604) -> ()
                n347 = Initialize Array(0.0 ("element"), w604, w607) -> (w606:dbl[][])
                n348 = local write "DelMatRul"(w606) -> ()
                n349 = local write "RulVarIdx"(w603) -> ()
              }
            }
            n350 = local read "Delta Matrix"() -> (w597:T2)
            n351 = Matrix Size(0:w597) -> (1:w596:i32)  [unwired: 1 out]
            n352 = Insert Into Array(array=w597, index (row)=0, new element=w598) -> (w599:T2)  [unwired: 1 in]
            "output array" <- w599
            n353 = local write "DelMatOrigSize"(w596) -> ()
            n354 = local write "Delta Matrix"(w599) -> ()
          }
          frame #6 {
            # "Performing Threshold Value Analysis"
            n355 = case shown="True" "Threshold Value Analysis" {
              frame False {
              }
              frame True {
                n356 = call "Threshold Value Settings.vi"() -> ("Threshold Value Settings 2"=w650:T9)  [unwired: 5 in]
                n357 = local read "Local Parameter Info"() -> (w645:string[][])
                n358 = local read "Idx of Mod in Sp IDs"() -> (w644:i32[])
                n359 = local read "Parameter info"() -> (w646:string[][])
                n360 = local read "ModTimeSym"() -> (w641:string)
                n361 = local read "Delta Matrix"() -> (w649:T2)
                n362 = local read "Species Info"() -> (w647:string[][])
                n363 = local read "CompSize"() -> (w642:string[])
                n364 = local read "Equations"() -> (w648:string[])
                n365 = local read "CompID"() -> (w643:string[])
                n366 = call "Search threshold value.vi"("Delta Matrix"=w649, "Idx of Mod in Sp IDs"=w644, "CompID"=w643, "CompSize"=w642, "Equations"=w648, "Species Info"=w647, "Parameter info"=w646, "Local Parameter Info"=w645, "Inputs"=w650, "ModTimeSym"=w641) -> ("Estimated T-delay"=w656:i32, "Th-High"=w655:dbl, "ET-Delay-SD"=w653:dbl, "E-OC-Th-High"=w654:dbl, "E-OC-Th-Low"=w651:dbl, "Th-Low"=w652:dbl)
                "Est Thresh Val" <- w655
                n367 = local read "Model Name"() -> (w638:string)
                n368 = local read "AppPath"() -> (w640:string)
                n369 = Concatenate Strings(w640, w638, "-TP-Analysis.txt") -> (w637:string)
                n370 = String To Path(string=w637) -> (path=w636:path)
                n371 = call "Threshold Results.vi"("Th-L-OC"=w651, "Th-Low"=w652, "file path (dialog if empty)"=w636, "Th-H-OC"=w654, "ET-Delay-SD"=w653, "Th-High"=w655, "Estimated Propagation Delay"=w656) -> ()  [unwired: 5 in]
              }
            }
          }
          frame #7 {
            n372 = local read "CompID"() -> (w659:string[])
            n373 = local read "Sp Ids"() -> (w658:string[])
            n374 = Build Array (concatenate)(string[] ["t"] ("array"), w658, w659) -> (w657:string[])
            n375 = local write "All Variables"(w657) -> ()
          }
          frame #8 {
            n376 = case shown="True" "Simulate SBML Events" {
              frame False {
              }
              frame True {
                n377 = local read "Events Info"() -> (w674:string[][])
                n378 = Index Array(array=w674, index (col)=6 ("disabled index (col)")) -> (element=w667:string[])  [unwired: 1 in]
                n379 = Index Array(array=w674, index (col)=7 ("disabled index (col)")) -> (element=w666:string[])  [unwired: 1 in]
                n380 = Index Array(array=w674, index (col)=4 ("disabled index (col)")) -> (element=w678:string[])  [unwired: 1 in]
                n381 = Index Array(array=w674, index (col)=5 ("disabled index (col)")) -> (element=w677:string[])  [unwired: 1 in]
                n382 = for {
                  tunnel: w678 -> [w706] mode=indexing
                  tunnel: [w696] -> w672 mode=indexing
                  tunnel: [w688] -> w663 mode=indexing
                  tunnel: [w698] -> w664 mode=indexing
                  tunnel: [w695] -> w662 mode=indexing
                  tunnel: w677 -> [w683] mode=indexing
                  tunnel: [w687] -> w671 mode=indexing
                  tunnel: [w686] -> w670 mode=indexing
                  tunnel: [w685] -> w669 mode=indexing
                  tunnel: [w684] -> w668 mode=indexing
                  n383 = Build Array(w683) -> (w682:string[])
                  n384 = call "Comma-separated-list extractor.vi"("In_list"=w682) -> ("List_Out"=w681:string[])  [unwired: 6 in, 1 out]
                  n385 = for {
                    tunnel: [w714] -> w687 mode=indexing
                    tunnel: [w713] -> w686 mode=indexing
                    tunnel: [w712] -> w685 mode=indexing
                    tunnel: [w711] -> w684 mode=indexing
                    tunnel: w681 -> [w707] mode=indexing
                    n386 = xnode "Match Regular Expression"("input string"=w707, "regular expression"="=") -> ("before match"=w719:string, "whole match"=w712:string, "after match"=w725:string)  [unwired: 4 in, 2 out]
                    n387 = call <vilib>:"Space Constant.vi"() -> ("String"=w723:string)
                    n388 = call <vilib>:"Space Constant.vi"() -> ("String"=w718:string)
                    n389 = Search and Replace String(input string=w725, search string=w723, replace string="") -> (result string=w708:string)  [unwired: 5 in, 3 out]
                    n390 = Search and Replace String(input string=w719, search string=w718, replace string="") -> (result string=w713:string)  [unwired: 5 in, 3 out]
                    n391 = local read "All Param Vals"() -> (w722:string[])
                    n392 = Search 1D Array(1D array=w722, element=w708) -> (index of element=w709:i32)  [unwired: 1 in]
                    n393 = case shown="1" w709 {
                      selector: w709 -> [_ w727]
                      tunnel: [w726 w728] -> w710
                      tunnel: w708 -> [w726 _]
                      frame 0, Default {
                      }
                      frame 1 {
                        n394 = local read "All Param Vals"() -> (w729:string[])
                        n395 = Index Array(array=w729, index=w727) -> (element=w728:string)
                      }
                    }
                    n396 = call <vilib>:"Space Constant.vi"() -> ("String"=w716:string)
                    n397 = Search and Replace String(input string=w710, search string=w716, replace string="") -> (result string=w711:string)  [unwired: 5 in, 3 out]
                    n398 = local read "All Variables"() -> (w721:string[])
                    n399 = Search 1D Array(1D array=w721, element=w713) -> (index of element=w714:i32)  [unwired: 1 in]
                  }
                  n400 = xnode "Match Regular Expression"("input string"=w706, "regular expression"="[><][=]|>|<") -> ("before match"=w704:string, "whole match"=w698:string, "after match"=w699:string)  [unwired: 4 in, 2 out]
                  n401 = call <vilib>:"Space Constant.vi"() -> ("String"=w701:string)
                  n402 = call <vilib>:"Space Constant.vi"() -> ("String"=w703:string)
                  n403 = Search and Replace String(input string=w699, search string=w701, replace string="") -> (result string=w690:string)  [unwired: 5 in, 3 out]
                  n404 = Search and Replace String(input string=w704, search string=w703, replace string="") -> (result string=w696:string)  [unwired: 5 in, 3 out]
                  n405 = local read "All Param IDs"() -> (w689:string[])
                  n406 = Search 1D Array(1D array=w689, element=w690) -> (index of element=w692:i32)  [unwired: 1 in]
                  n407 = case shown="0, Default" w692 {
                    selector: w692 -> [w845 _]
                    tunnel: [w844 w847] -> w691
                    tunnel: w690 -> [_ w847]
                    frame 0, Default {
                      n408 = local read "All Param Vals"() -> (w846:string[])
                      n409 = Index Array(array=w846, index=w845) -> (element=w844:string)
                    }
                    frame -1 {
                    }
                  }
                  n410 = call <vilib>:"Space Constant.vi"() -> ("String"=w694:string)
                  n411 = Search and Replace String(input string=w691, search string=w694, replace string="") -> (result string=w688:string)  [unwired: 5 in, 3 out]
                  n412 = local read "All Variables"() -> (w697:string[])
                  n413 = Search 1D Array(1D array=w697, element=w696) -> (index of element=w695:i32)  [unwired: 1 in]
                }
                "Var Idx" <- w662
                "Math Op" <- w664
                "Math Val" <- w663
                "Assign Val" <- w668
                "Assign Var Idx" <- w671
                n414 = Bundle By Name(cluster="Event Info", "Math Var"=w672, "Math Op"=w664, "Math Val"=w663, "Var Idx"=w662, "Assign Var Idx"=w671, "Assign Var"=w670, "Assign Op"=w669, "Assign Val"=w668, "Priority"=w667, "Delay"=w666) -> (w665:T1)
                n415 = local write "Event Info"(w665) -> ()
              }
            }
          }
          frame #9 {
            n416 = while {
              tunnel: [w1402] -> w962
              tunnel: w965 -> [w1411]
              i -> [w1416]
              stop <- w1412 stop-if-true
              # "after stop simulation everything is visible again"
              # "increase simulation speed"
              n417 = event shown="[2] \"Parameter info\", \"Local Parameter Info\", \"External Modifiers\": Value Change" {
                selector: _ -> [_ _ _]
                dyn-events: _ -> [_ _ _]
                timeout: 1 -> [_ _ _]
                tunnel: [w1440 w1570 w1820] -> w1414
                tunnel: [w1425 w1569 w1806] -> w1402
                event Timeout {
                  n418 = event-data() -> ()  [unwired: 1 in, 3 out]
                  n419 = local write "Boolean"(FALSE ("Boolean")) -> ()
                  n420 = stacked-sequence {
                    tunnel: [_ _ _ w1483 _ _ _ _ _ _ _] -> w1440
                    tunnel: [_ w1473 _ _ _ _ _ _ _ _ _] -> w1425
                    frame #0 {
                      n421 = local read "T"() -> (w1465:dbl[])
                      n422 = Array Size(array=w1465) -> (size(s)=w1464:i32)
                      n423 = Decrement(x=w1464) -> (x-1=w1463:i32)
                      n424 = Index Array(array=w1465, index=w1463) -> (element=w1457:dbl)
                      n425 = local read "Nxt Sp State (N)"() -> (w1460:dbl[])
                      n426 = local write "Nxt T"(w1457) -> ()
                      n427 = Insert Into Array(array=w1460, index=0, new element=w1457) -> (w1461:dbl[])
                      n428 = Equal?(x=w1457, y=inf) -> (x = y?=w1458:bool)
                      "T=inf" <- w1458
                      n429 = local write "Log Data"(w1461) -> ()
                      n430 = case shown="True" w1458 {
                        frame False {
                        }
                        frame True {
                          n431 = control-ref of="This VI"() -> (w1466:refnum<vi>)
                          n432 = invoke class="VI" method="FP.Close"(reference=w1466) -> (reference out=w1468:refnum<vi>, error out=w1467:errorcluster)  [unwired: 2 in, 1 out]
                          n433 = property on="Continous Simulation" class="Bool (strict)"("DisabledEnum"=T7."Enabled" ("Disabled")) -> ()  [unwired: 2 in, 2 out]
                          n434 = One Button Dialog(message="Next time of reaction is\ninfinity!\n\nVirtual instrument is closing.", button name ("OK")="Ok") -> (true=w1470:bool)
                          n435 = Close Reference(reference=w1468, error in (no error)=w1467) -> ()  [unwired: 1 out]
                          n436 = Stop(stop? (T)=w1470) -> ()
                        }
                      }
                    }
                    frame #1 {
                      n437 = local read "Log Data matrix"() -> (w1475:dbl[][])
                      n438 = local read "Log Data"() -> (w1474:dbl[])
                      n439 = Insert Into Array(array=w1475, new element=w1474) -> (w1473:dbl[][])  [unwired: 2 in]
                      n440 = local write "Log Data matrix"(w1473) -> ()
                    }
                    frame #2 {
                      n441 = disable-structure shown="Enabled" {
                        disable-tunnel: [w1481 w1482] -> w1479
                        frame Disabled {
                          n442 = local read "DataLog"() -> (w1480:path)
                          n443 = call-poly <vilib>:"Read From Spreadsheet File.vi"("file path (dialog if empty)"=w1480) -> ("all rows"=w1481:dbl[][])  [unwired: 6 in, 4 out]
                        }
                        frame Enabled {
                          n444 = local read "Log Data matrix"() -> (w1482:dbl[][])
                        }
                      }
                      n445 = Array Subset(array=w1479, index (row)=0 ("row 1"), index (col)=1 ("column 1")) -> (w1476:dbl[][])  [unwired: 2 in]
                      n446 = local write "Sp Data"(w1476) -> ()
                    }
                    frame #3 {
                      n447 = local read "Sp Data"() -> (w1485:dbl[][])
                      n448 = Transpose 2D Array(2D array=w1485) -> (transposed array=w1484:dbl[][])
                      n449 = for {
                        tunnel: w1484 -> [w1487] mode=indexing
                        tunnel: [w1486] -> w1483 mode=indexing
                        n450 = local read "T"() -> (w1488:dbl[])
                        n451 = Bundle("T"=w1488, w1487) -> (w1486:cluster{"T":dbl[], dbl[]})  [unwired: 1 in]
                      }
                    }
                    frame #4 {
                      n452 = local read "Nxt Sp State (N)"() -> (w1490:dbl[])
                      n453 = Number To Fractional String(number=w1490) -> (F-format string=w1489:string[])  [unwired: 3 in]
                      n454 = local write "Nxt Sp State (S)"(w1489) -> ()
                    }
                    frame #5 {
                      n455 = local read "All Param Names"() -> (w1500:string[])
                      n456 = local read "All Param Values"() -> (w1499:string[])
                      n457 = local read "Nxt Sp State (S)"() -> (w1497:string[])
                      n458 = local read "ModTimeSym"() -> (w1493:string)
                      n459 = local read "Equations"() -> (w1496:string[])
                      n460 = local read "CompSize"() -> (w1494:string[])
                      n461 = local read "CompID"() -> (w1495:string[])
                      n462 = local read "Sp Ids"() -> (w1498:string[])
                      n463 = local read "Nxt T"() -> (w1492:dbl)
                      n464 = Bundle By Name(cluster=T8 {"All Param Names"=["k1"], "All Param Values"=["1.5"], "Sp IDs"=["S1", "S2", "S3"], "Sp States"=["0.000000", "0.000000", "0.000000"], "Input Equations"=["C*k1*S1", "1.5*exp(time)^(-1)"], "CompID"=["C"], "CompSize"=["3.0"], "T-Sym"="time", "T"=0.0} ("Cluster"), "All Param Names"=w1500, "All Param Values"=w1499, "Sp IDs"=w1498, "Sp States"=w1497, "Input Equations"=w1496, "CompID"=w1495, "CompSize"=w1494, "T-Sym"=w1493, "T"=w1492) -> (w1502:T8)
                      n465 = call "Value substituter in equations.vi"("Cluster"=w1502) -> ("Output Equations"=w1503:string[])
                      n466 = for {
                        tunnel: w1503 -> [w1513] mode=indexing
                        tunnel: [w1509] -> w1504 mode=indexing
                        n467 = call <vilib>:"Eval Formula String.vi"("formula"=w1513) -> ("y value"=w1510:dbl)  [unwired: 1 in, 1 out]
                        n468 = In Range and Coerce(upper limit=inf, x=w1510, lower limit=0.0) -> (coerced(x)=w1509:dbl)  [unwired: 1 out]
                      }
                      n469 = local write "Output Equations"(w1503) -> ()
                      n470 = local write "Propensities"(w1504) -> ()
                      n471 = for {
                        tunnel: w1504 -> [w1508] mode=indexing
                        shift-right: [w1507] -> w1491
                        shift-left: 0.0 -> [w1506]
                        n472 = Add(x=w1506, y=w1508) -> (x+y=w1507:dbl)
                      }
                      n473 = local write "a0"(w1491) -> ()
                    }
                    frame #6 {
                      # "next time of reaction"
                      # "next reaction value"
                      n474 = Random Number (0-1)() -> (number: 0 to 1=w1515:dbl)
                      n475 = Random Number (0-1)() -> (number: 0 to 1=w1514:dbl)
                      n476 = local write "r1"(w1515) -> ()
                      n477 = local write "r2"(w1514) -> ()
                    }
                    frame #7 {
                      # "propensity is becoming zero.\nwhich makes Tau zero and thus time infinity"
                      # "(1/a0) * ln(1/r1)"
                      # "1/atot"
                      # "ln(1/r1)"
                      # "next reaction time"
                      n478 = local read "a0"() -> (w1524:dbl)
                      n479 = local read "r1"() -> (w1520:dbl)
                      n480 = Reciprocal(x=w1524) -> (1/x=w1522:dbl)
                      n481 = Reciprocal(x=w1520) -> (1/x=w1521:dbl)
                      n482 = Natural Logarithm(1:w1521) -> (0:w1523:dbl)
                      n483 = Compound Arithmetic op=MULTIPLY(w1522, w1523) -> (w1517:dbl)
                      n484 = In Range and Coerce(upper limit=inf, x=w1517, lower limit=0.0) -> (coerced(x)=w1516:dbl)  [unwired: 1 out]
                      n485 = local write "tau"(w1516) -> ()
                    }
                    frame #8 {
                      n486 = local read "L_cnt"() -> (w1537:i32)
                      n487 = local read "T"() -> (w1538:dbl[])
                      n488 = local read "a0"() -> (w1532:dbl)
                      n489 = local read "r2"() -> (w1531:dbl)
                      n490 = local read "tau"() -> (w1536:dbl)
                      n491 = Index Array(array=w1538, index=w1537) -> (element=w1535:dbl)
                      n492 = Multiply(x=w1532, y=w1531) -> (x*y=w1533:dbl)
                      n493 = local read "Continous Simulation"() -> (w1530:bool)
                      n494 = Add(x=w1535, y=w1536) -> (x+y=w1534:dbl)
                      n495 = local write "a0*r2"(w1533) -> ()
                      n496 = case shown="True" w1530 {
                        tunnel: w1534 -> [w1539 w1543]
                        tunnel: [w1539 w1540] -> w1525
                        frame False {
                        }
                        frame True {
                          n497 = local read "Time Limit"() -> (w1541:dbl)
                          n498 = In Range and Coerce(upper limit=w1541, x=w1543, lower limit=0.0) -> (coerced(x)=w1540:dbl)  [unwired: 1 out]
                        }
                      }
                      n499 = local read "L_cnt"() -> (w1527:i32)
                      n500 = local read "T"() -> (w1528:dbl[])
                      n501 = Increment(x=w1527) -> (x+1=w1526:i32)
                      n502 = Insert Into Array(array=w1528, index=w1526, new element=w1525) -> (w1529:dbl[])
                      n503 = local write "T"(w1529) -> ()
                    }
                    frame #9 {
                      # "Implement the selection of reaction algorithm"
                      n504 = local read "Propensities"() -> (w1545:dbl[])
                      n505 = for {
                        tunnel: w1545 -> [w1550] mode=indexing
                        shift-right: [w1548] -> _
                        shift-left: 0.0 -> [w1553]
                        i -> [w1546]
                        stop <- w1551 stop-if-true
                        n506 = Add(x=w1553, y=w1550) -> (x+y=w1548:dbl)
                        n507 = local read "a0*r2"() -> (w1549:dbl)
                        n508 = Greater?(x=w1548, y=w1549) -> (0:w1552:bool)
                        n509 = local write "Sum of Propensities for U"(w1548) -> ()
                        n510 = case shown="True" w1552 {
                          selector: w1552 -> [_ w1556]
                          tunnel: [w1554 w1556] -> w1551
                          tunnel: [w1554 w1556] -> w1547
                          tunnel: w1546 -> [_ w1555]
                          frame False {
                            w1554 = FALSE
                          }
                          frame True {
                            n511 = local write "Reac IDx"(w1555) -> ()
                          }
                        }
                        n512 = local write "Sum>a0*r2"(w1547) -> ()
                      }
                    }
                    frame #10 {
                      # "Extracting and adding the new state in the previous state of species"
                      n513 = local read "Delta Matrix"() -> (w1568:T2)
                      n514 = local read "Reac IDx"() -> (w1567:i32)
                      n515 = Index Array(array=w1568, index (row)=w1567) -> (element=w1566:T2)  [unwired: 1 in]
                      n516 = call-poly <vilib>:"Matrix To Array.vi"("Real Matrix"=w1566) -> ("Real 2D Array"=w1565:dbl[][])
                      n517 = local read "Nxt Sp State (N)"() -> (w1562:dbl[])
                      n518 = Transpose 2D Array(2D array=w1565) -> (transposed array=w1564:dbl[][])
                      n519 = Index Array(array=w1564, index (col)=0 ("disabled index (col)")) -> (element=w1561:dbl[])  [unwired: 1 in]
                      n520 = Add(x=w1561, y=w1562) -> (x+y=w1560:dbl[])
                      n521 = local write "Reac to execute"(w1561) -> ()
                      n522 = In Range and Coerce(upper limit=inf, x=w1560, lower limit=0.0) -> (coerced(x)=w1557:dbl[])  [unwired: 1 out]
                      n523 = local write "Nxt Sp State (N)"(w1557) -> ()
                    }
                  }
                  n524 = Index Array(array="Parameter info", index (col)=0 ("disabled index (col)")) -> (element=w1434:string[])  [unwired: 1 in]
                  n525 = Index Array(array="Parameter info", index (col)=2 ("disabled index (col)")) -> (element=w1432:string[])  [unwired: 1 in]
                  n526 = Index Array(array="Local Parameter Info", index (col)=0 ("disabled index (col)")) -> (element=w1433:string[])  [unwired: 1 in]
                  n527 = Index Array(array="Local Parameter Info", index (col)=1 ("disabled index (col)")) -> (element=w1431:string[])  [unwired: 1 in]
                  n528 = Insert Into Array(array=w1432, new element=w1431) -> (w1427:string[])  [unwired: 1 in]
                  n529 = Insert Into Array(array=w1434, new element=w1433) -> (w1428:string[])  [unwired: 1 in]
                  n530 = local write "All Param Names"(w1428) -> ()
                  n531 = local write "All Param Values"(w1427) -> ()
                  n532 = local read "Trig  MSW"() -> (w1426:bool)
                  n533 = case shown="True" w1426 {
                    tunnel: w1425 -> [_ w1441]
                    frame False {
                    }
                    frame True {
                      n534 = local read "DataLog"() -> (w1442:path)
                      n535 = stacked-sequence {
                        tunnel: w1442 -> [w1444 _ w1450 _ w1454]
                        tunnel: w1441 -> [_ _ w1449 _ _]
                        frame #0 {
                          n536 = local read "Sp Ids"() -> (w1443:string[])
                          n537 = Insert Into Array(array=w1443, index=0, new element="Time" ("string")) -> (w1447:string[])
                          n538 = call-poly <vilib>:"Write To Spreadsheet File.vi"("1D data"=w1447, "file path (dialog if empty)"=w1444) -> ()  [unwired: 6 in, 1 out]
                        }
                        frame #1 {
                          n539 = Wait (ms)(milliseconds to wait=u32 3) -> ()  [unwired: 1 out]
                        }
                        frame #2 {
                          n540 = call-poly <vilib>:"Write To Spreadsheet File.vi"("append to file? (new file:F)"=TRUE, "2D data"=w1449, "file path (dialog if empty)"=w1450) -> ()  [unwired: 5 in, 1 out]
                        }
                        frame #3 {
                          n541 = Wait (ms)(milliseconds to wait=u32 3) -> ()  [unwired: 1 out]
                        }
                        frame #4 {
                          n542 = local read "Est Thresh Val"() -> (w1455:dbl)
                          n543 = local read "Plot colors"() -> (w1453:u32[])
                          n544 = call "Test_Dig_Wfm.vi"("Plot Colors"=w1453, "Threshold Value of a circuit"=w1455, "DataLog"=w1454) -> ("Close 2"=w1456:bool)  [unwired: 8 in]
                          n545 = local write "Trig  MSW"(w1456) -> ()
                        }
                      }
                    }
                  }
                }
                event "Logic Verification": Value Change {
                  n546 = event-data() -> ()  [unwired: 1 in, 6 out]
                  n547 = case shown="False" "Logic Verification" {
                    tunnel: [w1573 w1681] -> w1570
                    tunnel: [w1572 w1680] -> w1569
                    frame False {
                      n548 = stacked-sequence {
                        tunnel: [_ _ _ w1597 _ _ _ _ _ _ _] -> w1573
                        tunnel: [_ w1587 _ _ _ _ _ _ _ _ _] -> w1572
                        frame #0 {
                          n549 = local read "T"() -> (w1582:dbl[])
                          n550 = Array Size(array=w1582) -> (size(s)=w1581:i32)
                          n551 = Decrement(x=w1581) -> (x-1=w1580:i32)
                          n552 = Index Array(array=w1582, index=w1580) -> (element=w1575:dbl)
                          n553 = local read "Nxt Sp State (N)"() -> (w1577:dbl[])
                          n554 = local write "Nxt T"(w1575) -> ()
                          n555 = Insert Into Array(array=w1577, index=0, new element=w1575) -> (w1578:dbl[])
                          n556 = Equal?(x=w1575, y=inf) -> (x = y?=w1574:bool)
                          n557 = local write "Log Data"(w1578) -> ()
                          n558 = local write "T=inf"(w1574) -> ()
                          n559 = case shown="True" w1574 {
                            frame False {
                            }
                            frame True {
                              n560 = property on="Continous Simulation" class="Bool (strict)"("DisabledEnum"=T7."Enabled" ("Disabled")) -> ()  [unwired: 2 in, 2 out]
                              n561 = One Button Dialog(message="Next time of reaction is\ninfinity!", button name ("OK")="Ok") -> (true=w1584:bool)
                              n562 = Stop(stop? (T)=w1584) -> ()
                            }
                          }
                        }
                        frame #1 {
                          n563 = local read "Log Data matrix"() -> (w1589:dbl[][])
                          n564 = local read "Log Data"() -> (w1588:dbl[])
                          n565 = Insert Into Array(array=w1589, new element=w1588) -> (w1587:dbl[][])  [unwired: 2 in]
                          n566 = local write "Log Data matrix"(w1587) -> ()
                        }
                        frame #2 {
                          n567 = disable-structure shown="Enabled" {
                            disable-tunnel: [w1595 w1596] -> w1593
                            frame Disabled {
                              n568 = local read "DataLog"() -> (w1594:path)
                              n569 = call-poly <vilib>:"Read From Spreadsheet File.vi"("file path (dialog if empty)"=w1594) -> ("all rows"=w1595:dbl[][])  [unwired: 6 in, 4 out]
                            }
                            frame Enabled {
                              n570 = local read "Log Data matrix"() -> (w1596:dbl[][])
                            }
                          }
                          n571 = Array Subset(array=w1593, index (row)=0 ("row 1"), index (col)=1 ("column 1")) -> (w1590:dbl[][])  [unwired: 2 in]
                          n572 = local write "Sp Data"(w1590) -> ()
                        }
                        frame #3 {
                          n573 = local read "Sp Data"() -> (w1599:dbl[][])
                          n574 = Transpose 2D Array(2D array=w1599) -> (transposed array=w1598:dbl[][])
                          n575 = for {
                            tunnel: w1598 -> [w1601] mode=indexing
                            tunnel: [w1600] -> w1597 mode=indexing
                            n576 = local read "T"() -> (w1602:dbl[])
                            n577 = Bundle("T"=w1602, w1601) -> (w1600:cluster{"T":dbl[], dbl[]})  [unwired: 1 in]
                          }
                        }
                        frame #4 {
                          n578 = local read "Nxt Sp State (N)"() -> (w1604:dbl[])
                          n579 = Number To Fractional String(number=w1604) -> (F-format string=w1603:string[])  [unwired: 3 in]
                          n580 = local write "Nxt Sp State (S)"(w1603) -> ()
                        }
                        frame #5 {
                          n581 = local read "All Param Names"() -> (w1615:string[])
                          n582 = local read "All Param Values"() -> (w1614:string[])
                          n583 = local read "Nxt Sp State (S)"() -> (w1612:string[])
                          n584 = local read "ModTimeSym"() -> (w1608:string)
                          n585 = local read "Equations"() -> (w1611:string[])
                          n586 = local read "CompSize"() -> (w1609:string[])
                          n587 = local read "CompID"() -> (w1610:string[])
                          n588 = local read "Sp Ids"() -> (w1613:string[])
                          n589 = local read "Nxt T"() -> (w1607:dbl)
                          n590 = Bundle By Name(cluster=T8 {"All Param Names"=["k1"], "All Param Values"=["1.5"], "Sp IDs"=["S1", "S2", "S3"], "Sp States"=["0.000000", "0.000000", "0.000000"], "Input Equations"=["C*k1*S1", "1.5*exp(time)^(-1)"], "CompID"=["C"], "CompSize"=["3.0"], "T-Sym"="time", "T"=0.0} ("Cluster"), "All Param Names"=w1615, "All Param Values"=w1614, "Sp IDs"=w1613, "Sp States"=w1612, "Input Equations"=w1611, "CompID"=w1610, "CompSize"=w1609, "T-Sym"=w1608, "T"=w1607) -> (w1617:T8)
                          n591 = call "Value substituter in equations.vi"("Cluster"=w1617) -> ("Output Equations"=w1606:string[])
                          n592 = local write "Output Equations"(w1606) -> ()
                          n593 = for {
                            tunnel: w1606 -> [w1624] mode=indexing
                            tunnel: [w1620] -> w1605 mode=indexing
                            n594 = call <vilib>:"Eval Formula String.vi"("formula"=w1624) -> ("y value"=w1621:dbl)  [unwired: 1 in, 1 out]
                            n595 = In Range and Coerce(upper limit=inf, x=w1621, lower limit=0.0) -> (coerced(x)=w1620:dbl)  [unwired: 1 out]
                          }
                          n596 = local write "Propensities"(w1605) -> ()
                          n597 = for {
                            tunnel: w1605 -> [w1627] mode=indexing
                            shift-right: [w1626] -> w1618
                            shift-left: 0.0 -> [w1625]
                            n598 = Add(x=w1625, y=w1627) -> (x+y=w1626:dbl)
                          }
                          n599 = local write "a0"(w1618) -> ()
                        }
                        frame #6 {
                          # "next time of reaction"
                          # "next reaction value"
                          n600 = Random Number (0-1)() -> (number: 0 to 1=w1629:dbl)
                          n601 = Random Number (0-1)() -> (number: 0 to 1=w1628:dbl)
                          n602 = local write "r1"(w1629) -> ()
                          n603 = local write "r2"(w1628) -> ()
                        }
                        frame #7 {
                          # "propensity is becoming zero.\nwhich makes Tau zero and thus time infinity"
                          # "(1/a0) * ln(1/r1)"
                          # "1/atot"
                          # "ln(1/r1)"
                          # "next reaction time"
                          n604 = local read "a0"() -> (w1635:dbl)
                          n605 = local read "r1"() -> (w1630:dbl)
                          n606 = Reciprocal(x=w1635) -> (1/x=w1632:dbl)
                          n607 = Reciprocal(x=w1630) -> (1/x=w1631:dbl)
                          n608 = Natural Logarithm(1:w1631) -> (0:w1633:dbl)
                          n609 = Compound Arithmetic op=MULTIPLY(w1632, w1633) -> (w1634:dbl)
                          n610 = local write "tau"(w1634) -> ()
                        }
                        frame #8 {
                          n611 = local read "L_cnt"() -> (w1648:i32)
                          n612 = local read "T"() -> (w1649:dbl[])
                          n613 = local read "a0"() -> (w1643:dbl)
                          n614 = local read "r2"() -> (w1642:dbl)
                          n615 = local read "tau"() -> (w1647:dbl)
                          n616 = Index Array(array=w1649, index=w1648) -> (element=w1646:dbl)
                          n617 = Multiply(x=w1643, y=w1642) -> (x*y=w1644:dbl)
                          n618 = local read "Continous Simulation"() -> (w1641:bool)
                          n619 = Add(x=w1646, y=w1647) -> (x+y=w1645:dbl)
                          n620 = local write "a0*r2"(w1644) -> ()
                          n621 = case shown="True" w1641 {
                            tunnel: w1645 -> [w1650 w1654]
                            tunnel: [w1650 w1651] -> w1636
                            frame False {
                            }
                            frame True {
                              n622 = local read "Time Limit"() -> (w1652:dbl)
                              n623 = In Range and Coerce(upper limit=w1652, x=w1654, lower limit=0.0) -> (coerced(x)=w1651:dbl)  [unwired: 1 out]
                            }
                          }
                          n624 = local read "L_cnt"() -> (w1638:i32)
                          n625 = local read "T"() -> (w1639:dbl[])
                          n626 = Increment(x=w1638) -> (x+1=w1637:i32)
                          n627 = Insert Into Array(array=w1639, index=w1637, new element=w1636) -> (w1640:dbl[])
                          n628 = local write "T"(w1640) -> ()
                        }
                        frame #9 {
                          # "Implement the selection of reaction algorithm"
                          n629 = local read "Propensities"() -> (w1656:dbl[])
                          n630 = for {
                            tunnel: w1656 -> [w1661] mode=indexing
                            shift-right: [w1659] -> _
                            shift-left: 0.0 -> [w1664]
                            i -> [w1657]
                            stop <- w1662 stop-if-true
                            n631 = Add(x=w1664, y=w1661) -> (x+y=w1659:dbl)
                            n632 = local read "a0*r2"() -> (w1660:dbl)
                            n633 = Greater?(x=w1659, y=w1660) -> (0:w1663:bool)
                            n634 = local write "Sum of Propensities for U"(w1659) -> ()
                            n635 = case shown="True" w1663 {
                              selector: w1663 -> [_ w1667]
                              tunnel: [w1665 w1667] -> w1662
                              tunnel: [w1665 w1667] -> w1658
                              tunnel: w1657 -> [_ w1666]
                              frame False {
                                w1665 = FALSE
                              }
                              frame True {
                                n636 = local write "Reac IDx"(w1666) -> ()
                              }
                            }
                            n637 = local write "Sum>a0*r2"(w1658) -> ()
                          }
                        }
                        frame #10 {
                          # "Extracting and adding the new state in the previous state of species"
                          n638 = local read "Delta Matrix"() -> (w1679:T2)
                          n639 = local read "Reac IDx"() -> (w1678:i32)
                          n640 = Index Array(array=w1679, index (row)=w1678) -> (element=w1677:T2)  [unwired: 1 in]
                          n641 = call-poly <vilib>:"Matrix To Array.vi"("Real Matrix"=w1677) -> ("Real 2D Array"=w1676:dbl[][])
                          n642 = local read "Nxt Sp State (N)"() -> (w1673:dbl[])
                          n643 = Transpose 2D Array(2D array=w1676) -> (transposed array=w1675:dbl[][])
                          n644 = Index Array(array=w1675, index (col)=0 ("disabled index (col)")) -> (element=w1672:dbl[])  [unwired: 1 in]
                          n645 = Add(x=w1672, y=w1673) -> (x+y=w1671:dbl[])
                          n646 = local write "Reac to execute"(w1672) -> ()
                          n647 = In Range and Coerce(upper limit=inf, x=w1671, lower limit=0.0) -> (coerced(x)=w1668:dbl[])  [unwired: 1 out]
                          n648 = local write "Nxt Sp State (N)"(w1668) -> ()
                        }
                      }
                    }
                    frame True {
                      n649 = stacked-sequence {
                        tunnel: [_ _ _ _ _ _ w1724 _ _ _ _ _ _ _] -> w1681
                        tunnel: [_ _ _ _ w1713 _ _ _ _ _ _ _ _ _] -> w1680
                        frame #0 {
                          n650 = local read "Log Data matrix"() -> (w1682:dbl[][])
                          n651 = local read "DataLog"() -> (w1683:path)
                          n652 = call-poly <vilib>:"Write To Spreadsheet File.vi"("append to file? (new file:F)"=TRUE, "2D data"=w1682, "file path (dialog if empty)"=w1683) -> ()  [unwired: 5 in, 1 out]
                        }
                        frame #1 {
                          n653 = local read "Threshold Value Analysis"() -> (w1686:bool)
                          n654 = local read "Est Thresh Val"() -> (w1685:dbl)
                          n655 = local read "Model Name"() -> (w1687:string)
                          n656 = local read "Ex_Mod_IDs"() -> (w1688:string[])
                          n657 = local read "Sp Ids"() -> (w1689:string[])
                          n658 = call "BLE v2.0-scalable.vi"("Est Thresh Val"=w1685, "Threshold Value Analysis"=w1686, "Model Name"=w1687, "Ex_Mod_IDs"=w1688, "Sp_Id_Arr"=w1689) -> ()  [unwired: 5 in, 2 out]
                        }
                        frame #2 {
                          n659 = local read "External Modifiers"() -> (w1690:T3[])
                          n660 = local read "Idx of Mod in Sp IDs"() -> (w1691:i32[])
                          n661 = for {
                            tunnel: w1691 -> [w1695] mode=indexing
                            tunnel: w1690 -> [w1693] mode=indexing
                            n662 = Unbundle By Name(w1693) -> ("Dial"=w1692:dbl)
                            n663 = local read "Nxt Sp State (N)"() -> (w1696:dbl[])
                            n664 = Replace Array Subset(array=w1696, new element=w1692, index=w1695) -> (w1694:dbl[])
                            n665 = local write "Nxt Sp State (N)"(w1694) -> ()
                          }
                        }
                        frame #3 {
                          n666 = local read "T"() -> (w1698:dbl[])
                          n667 = Array Size(array=w1698) -> (size(s)=w1699:i32)
                          n668 = Decrement(x=w1699) -> (x-1=w1700:i32)
                          n669 = Index Array(array=w1698, index=w1700) -> (element=w1705:dbl)
                          n670 = local read "Nxt Sp State (N)"() -> (w1703:dbl[])
                          n671 = Insert Into Array(array=w1703, index=0, new element=w1705) -> (w1702:dbl[])
                          n672 = local write "Nxt T"(w1705) -> ()
                          n673 = local write "Log Data"(w1702) -> ()
                          n674 = Equal?(x=w1705, y=inf) -> (x = y?=w1697:bool)
                          n675 = local write "T=inf"(w1697) -> ()
                          n676 = case shown="True" w1697 {
                            frame False {
                            }
                            frame True {
                              n677 = control-ref of="This VI"() -> (w1706:refnum<vi>)
                              n678 = invoke class="VI" method="FP.Close"(reference=w1706) -> (reference out=w1708:refnum<vi>, error out=w1707:errorcluster)  [unwired: 2 in, 1 out]
                              n679 = property on="Continous Simulation" class="Bool (strict)"("DisabledEnum"=T7."Enabled" ("Disabled")) -> ()  [unwired: 2 in, 2 out]
                              n680 = One Button Dialog(message="Next time of reaction is\ninfinity!\n\nVirtual instrument is closing.", button name ("OK")="Ok") -> (true=w1710:bool)
                              n681 = Close Reference(reference=w1708, error in (no error)=w1707) -> ()  [unwired: 1 out]
                              n682 = Stop(stop? (T)=w1710) -> ()
                            }
                          }
                        }
                        frame #4 {
                          n683 = local read "Log Data matrix"() -> (w1715:dbl[][])
                          n684 = local read "Log Data"() -> (w1714:dbl[])
                          n685 = Insert Into Array(array=w1715, new element=w1714) -> (w1713:dbl[][])  [unwired: 2 in]
                          n686 = local write "Log Data matrix"(w1713) -> ()
                        }
                        frame #5 {
                          n687 = disable-structure shown="Enabled" {
                            disable-tunnel: [w1721 w1722] -> w1719
                            frame Disabled {
                              n688 = local read "DataLog"() -> (w1720:path)
                              n689 = call-poly <vilib>:"Read From Spreadsheet File.vi"("file path (dialog if empty)"=w1720) -> ("all rows"=w1721:dbl[][])  [unwired: 6 in, 4 out]
                            }
                            frame Enabled {
                              n690 = local read "Log Data matrix"() -> (w1722:dbl[][])
                            }
                          }
                          n691 = Array Subset(array=w1719, index (row)=1 ("row 1"), index (col)=1 ("column 1")) -> (w1716:dbl[][])  [unwired: 2 in]
                          n692 = local write "Sp Data"(w1716) -> ()
                        }
                        frame #6 {
                          n693 = local read "Sp Data"() -> (w1725:dbl[][])
                          n694 = Transpose 2D Array(2D array=w1725) -> (transposed array=w1723:dbl[][])
                          n695 = for {
                            tunnel: w1723 -> [w1726] mode=indexing
                            tunnel: [w1727] -> w1724 mode=indexing
                            n696 = local read "T"() -> (w1728:dbl[])
                            n697 = Bundle("T"=w1728, w1726) -> (w1727:cluster{"T":dbl[], dbl[]})  [unwired: 1 in]
                          }
                        }
                        frame #7 {
                          n698 = local read "Nxt Sp State (N)"() -> (w1730:dbl[])
                          n699 = Number To Fractional String(number=w1730) -> (F-format string=w1729:string[])  [unwired: 3 in]
                          n700 = local write "Nxt Sp State (S)"(w1729) -> ()
                        }
                        frame #8 {
                          n701 = local read "All Param Names"() -> (w1733:string[])
                          n702 = local read "All Param Values"() -> (w1734:string[])
                          n703 = local read "Nxt Sp State (S)"() -> (w1736:string[])
                          n704 = local read "ModTimeSym"() -> (w1740:string)
                          n705 = local read "Equations"() -> (w1737:string[])
                          n706 = local read "CompSize"() -> (w1739:string[])
                          n707 = local read "CompID"() -> (w1738:string[])
                          n708 = local read "Sp Ids"() -> (w1735:string[])
                          n709 = local read "Nxt T"() -> (w1741:dbl)
                          n710 = Bundle By Name(cluster=T8 {"All Param Names"=["k1"], "All Param Values"=["1.5"], "Sp IDs"=["S1", "S2", "S3"], "Sp States"=["0.000000", "0.000000", "0.000000"], "Input Equations"=["C*k1*S1", "1.5*exp(time)^(-1)"], "CompID"=["C"], "CompSize"=["3.0"], "T-Sym"="time", "T"=0.0} ("Cluster"), "All Param Names"=w1733, "All Param Values"=w1734, "Sp IDs"=w1735, "Sp States"=w1736, "Input Equations"=w1737, "CompID"=w1738, "CompSize"=w1739, "T-Sym"=w1740, "T"=w1741) -> (w1731:T8)
                          n711 = call "Value substituter in equations.vi"("Cluster"=w1731) -> ("Output Equations"=w1742:string[])
                          n712 = for {
                            tunnel: w1742 -> [w1753] mode=indexing
                            tunnel: [w1749] -> w1744 mode=indexing
                            n713 = call <vilib>:"Eval Formula String.vi"("formula"=w1753) -> ("y value"=w1750:dbl)  [unwired: 1 in, 1 out]
                            n714 = In Range and Coerce(upper limit=inf, x=w1750, lower limit=0.0) -> (coerced(x)=w1749:dbl)  [unwired: 1 out]
                          }
                          n715 = local write "Output Equations"(w1742) -> ()
                          n716 = for {
                            tunnel: w1744 -> [w1748] mode=indexing
                            shift-right: [w1747] -> w1743
                            shift-left: 0.0 -> [w1746]
                            n717 = Add(x=w1746, y=w1748) -> (x+y=w1747:dbl)
                          }
                          n718 = local write "Propensities"(w1744) -> ()
                          n719 = local write "a0"(w1743) -> ()
                        }
                        frame #9 {
                          # "next time of reaction"
                          # "next reaction value"
                          n720 = Random Number (0-1)() -> (number: 0 to 1=w1755:dbl)
                          n721 = Random Number (0-1)() -> (number: 0 to 1=w1754:dbl)
                          n722 = local write "r1"(w1755) -> ()
                          n723 = local write "r2"(w1754) -> ()
                        }
                        frame #10 {
                          # "(1/a0) * ln(1/r1)"
                          # "1/atot"
                          # "ln(1/r1)"
                          # "next reaction time"
                          n724 = local read "a0"() -> (w1761:dbl)
                          n725 = local read "r1"() -> (w1756:dbl)
                          n726 = Reciprocal(x=w1761) -> (1/x=w1758:dbl)
                          n727 = Reciprocal(x=w1756) -> (1/x=w1757:dbl)
                          n728 = Natural Logarithm(1:w1757) -> (0:w1759:dbl)
                          n729 = Compound Arithmetic op=MULTIPLY(w1758, w1759) -> (w1760:dbl)
                          n730 = local write "tau"(w1760) -> ()
                        }
                        frame #11 {
                          n731 = local read "L_cnt"() -> (w1763:i32)
                          n732 = local read "Continous Simulation"() -> (w1770:bool)
                          n733 = local read "T"() -> (w1762:dbl[])
                          n734 = local read "tau"() -> (w1764:dbl)
                          n735 = Index Array(array=w1762, index=w1763) -> (element=w1765:dbl)
                          n736 = Add(x=w1765, y=w1764) -> (x+y=w1766:dbl)
                          n737 = case shown="True" w1770 {
                            tunnel: w1766 -> [w1776 w1780]
                            tunnel: [w1776 w1777] -> w1775
                            frame False {
                            }
                            frame True {
                              n738 = local read "Time Limit"() -> (w1778:dbl)
                              n739 = In Range and Coerce(upper limit=w1778, x=w1780, lower limit=0.0) -> (coerced(x)=w1777:dbl)  [unwired: 1 out]
                            }
                          }
                          n740 = local read "L_cnt"() -> (w1773:i32)
                          n741 = Increment(x=w1773) -> (x+1=w1774:i32)
                          n742 = local read "T"() -> (w1772:dbl[])
                          n743 = local read "a0"() -> (w1768:dbl)
                          n744 = local read "r2"() -> (w1769:dbl)
                          n745 = Insert Into Array(array=w1772, index=w1774, new element=w1775) -> (w1771:dbl[])
                          n746 = Multiply(x=w1768, y=w1769) -> (x*y=w1767:dbl)
                          n747 = local write "T"(w1771) -> ()
                          n748 = local write "a0*r2"(w1767) -> ()
                        }
                        frame #12 {
                          # "Implement the selection of reaction algorithm"
                          n749 = local read "Propensities"() -> (w1782:dbl[])
                          n750 = for {
                            tunnel: w1782 -> [w1787] mode=indexing
                            shift-right: [w1785] -> _
                            shift-left: 0.0 -> [w1790]
                            i -> [w1783]
                            stop <- w1788 stop-if-true
                            n751 = local read "a0*r2"() -> (w1786:dbl)
                            n752 = Add(x=w1790, y=w1787) -> (x+y=w1785:dbl)
                            n753 = Greater?(x=w1785, y=w1786) -> (0:w1789:bool)
                            n754 = local write "Sum of Propensities for U"(w1785) -> ()
                            n755 = case shown="True" w1789 {
                              selector: w1789 -> [_ w1793]
                              tunnel: [w1791 w1793] -> w1788
                              tunnel: [w1791 w1793] -> w1784
                              tunnel: w1783 -> [_ w1792]
                              frame False {
                                w1791 = FALSE
                              }
                              frame True {
                                n756 = local write "Reac IDx"(w1792) -> ()
                              }
                            }
                            n757 = local write "Sum>a0*r2"(w1784) -> ()
                          }
                        }
                        frame #13 {
                          # "Extracting and adding the new state in the previous state of species"
                          n758 = local read "Delta Matrix"() -> (w1794:T2)
                          n759 = local read "Reac IDx"() -> (w1795:i32)
                          n760 = Index Array(array=w1794, index (row)=w1795) -> (element=w1796:T2)  [unwired: 1 in]
                          n761 = call-poly <vilib>:"Matrix To Array.vi"("Real Matrix"=w1796) -> ("Real 2D Array"=w1797:dbl[][])
                          n762 = local read "Nxt Sp State (N)"() -> (w1800:dbl[])
                          n763 = Transpose 2D Array(2D array=w1797) -> (transposed array=w1798:dbl[][])
                          n764 = Index Array(array=w1798, index (col)=0 ("disabled index (col)")) -> (element=w1801:dbl[])  [unwired: 1 in]
                          n765 = Add(x=w1801, y=w1800) -> (x+y=w1802:dbl[])
                          n766 = local write "Reac to execute"(w1801) -> ()
                          n767 = In Range and Coerce(upper limit=inf, x=w1802, lower limit=0.0) -> (coerced(x)=w1805:dbl[])  [unwired: 1 out]
                          n768 = local write "Nxt Sp State (N)"(w1805) -> ()
                        }
                      }
                    }
                  }
                }
                event "Parameter info", "Local Parameter Info", "External Modifiers": Value Change {
                  n769 = event-data() -> ()  [unwired: 1 in, 6 out]
                  n770 = local read "Local Parameter Info"() -> (w1809:string[][])
                  n771 = local write "Boolean"(TRUE ("Boolean")) -> ()
                  n772 = local read "Parameter info"() -> (w1810:string[][])
                  n773 = Index Array(array=w1810, index (col)=0 ("disabled index (col)")) -> (element=w1814:string[])  [unwired: 1 in]
                  n774 = Index Array(array=w1810, index (col)=2 ("disabled index (col)")) -> (element=w1812:string[])  [unwired: 1 in]
                  n775 = Index Array(array=w1809, index (col)=0 ("disabled index (col)")) -> (element=w1813:string[])  [unwired: 1 in]
                  n776 = Index Array(array=w1809, index (col)=1 ("disabled index (col)")) -> (element=w1811:string[])  [unwired: 1 in]
                  n777 = Insert Into Array(array=w1814, new element=w1813) -> (w1808:string[])  [unwired: 1 in]
                  n778 = Insert Into Array(array=w1812, new element=w1811) -> (w1807:string[])  [unwired: 1 in]
                  n779 = stacked-sequence {
                    tunnel: [_ _ _ _ w1854 _ _ _ _ _ _ _] -> w1820
                    tunnel: w1807 -> [_ _ _ _ _ _ _ _ _ _ _ _]
                    tunnel: [_ _ w1844 _ _ _ _ _ _ _ _ _] -> w1806
                    frame #0 {
                      n780 = local read "Idx of Mod in Sp IDs"() -> (w1822:i32[])
                      n781 = local read "External Modifiers"() -> (w1821:T3[])
                      n782 = for {
                        tunnel: w1822 -> [w1826] mode=indexing
                        tunnel: w1821 -> [w1824] mode=indexing
                        n783 = Unbundle By Name(w1824) -> ("Dial"=w1823:dbl)
                        n784 = local read "Nxt Sp State (N)"() -> (w1827:dbl[])
                        n785 = Replace Array Subset(array=w1827, new element=w1823, index=w1826) -> (w1825:dbl[])
                        n786 = local write "Nxt Sp State (N)"(w1825) -> ()
                      }
                    }
                    frame #1 {
                      n787 = local read "T"() -> (w1829:dbl[])
                      n788 = Array Size(array=w1829) -> (size(s)=w1830:i32)
                      n789 = Decrement(x=w1830) -> (x-1=w1831:i32)
                      n790 = Index Array(array=w1829, index=w1831) -> (element=w1836:dbl)
                      n791 = local read "Nxt Sp State (N)"() -> (w1834:dbl[])
                      n792 = Insert Into Array(array=w1834, index=0, new element=w1836) -> (w1833:dbl[])
                      n793 = local write "Nxt T"(w1836) -> ()
                      n794 = local write "Log Data"(w1833) -> ()
                      n795 = Equal?(x=w1836, y=inf) -> (x = y?=w1828:bool)
                      n796 = local write "T=inf"(w1828) -> ()
                      n797 = case shown="True" w1828 {
                        frame False {
                        }
                        frame True {
                          n798 = control-ref of="This VI"() -> (w1839:refnum<vi>)
                          n799 = invoke class="VI" method="FP.Close"(reference=w1839) -> (reference out=w1837:refnum<vi>, error out=w1838:errorcluster)  [unwired: 2 in, 1 out]
                          n800 = property on="Continous Simulation" class="Bool (strict)"("DisabledEnum"=T7."Enabled" ("Disabled")) -> ()  [unwired: 2 in, 2 out]
                          n801 = One Button Dialog(message="Next time of reaction is\ninfinity!\n\nVirtual instrument is closing.", button name ("OK")="Ok") -> (true=w1841:bool)
                          n802 = Close Reference(reference=w1837, error in (no error)=w1838) -> ()  [unwired: 1 out]
                          n803 = Stop(stop? (T)=w1841) -> ()
                        }
                      }
                    }
                    frame #2 {
                      n804 = local read "Log Data matrix"() -> (w1846:dbl[][])
                      n805 = local read "Log Data"() -> (w1845:dbl[])
                      n806 = Insert Into Array(array=w1846, new element=w1845) -> (w1844:dbl[][])  [unwired: 2 in]
                      n807 = local write "Log Data matrix"(w1844) -> ()
                    }
                    frame #3 {
                      n808 = disable-structure shown="Enabled" {
                        disable-tunnel: [w1852 w1853] -> w1850
                        frame Disabled {
                          n809 = local read "DataLog"() -> (w1851:path)
                          n810 = call-poly <vilib>:"Read From Spreadsheet File.vi"("file path (dialog if empty)"=w1851) -> ("all rows"=w1852:dbl[][])  [unwired: 6 in, 4 out]
                        }
                        frame Enabled {
                          n811 = local read "Log Data matrix"() -> (w1853:dbl[][])
                        }
                      }
                      n812 = Array Subset(array=w1850, index (row)=1 ("row 1"), index (col)=1 ("column 1")) -> (w1847:dbl[][])  [unwired: 2 in]
                      n813 = local write "Sp Data"(w1847) -> ()
                    }
                    frame #4 {
                      n814 = local read "Sp Data"() -> (w1856:dbl[][])
                      n815 = Transpose 2D Array(2D array=w1856) -> (transposed array=w1855:dbl[][])
                      n816 = for {
                        tunnel: w1855 -> [w1858] mode=indexing
                        tunnel: [w1857] -> w1854 mode=indexing
                        n817 = local read "T"() -> (w1859:dbl[])
                        n818 = Bundle("T"=w1859, w1858) -> (w1857:cluster{"T":dbl[], dbl[]})  [unwired: 1 in]
                      }
                    }
                    frame #5 {
                      n819 = local read "Nxt Sp State (N)"() -> (w1861:dbl[])
                      n820 = Number To Fractional String(number=w1861) -> (F-format string=w1860:string[])  [unwired: 3 in]
                      n821 = local write "Nxt Sp State (S)"(w1860) -> ()
                    }
                    frame #6 {
                      n822 = local read "All Param Names"() -> (w1871:string[])
                      n823 = local read "All Param Values"() -> (w1870:string[])
                      n824 = local read "Nxt Sp State (S)"() -> (w1868:string[])
                      n825 = local read "ModTimeSym"() -> (w1864:string)
                      n826 = local read "Equations"() -> (w1867:string[])
                      n827 = local read "CompSize"() -> (w1865:string[])
                      n828 = local read "CompID"() -> (w1866:string[])
                      n829 = local read "Sp Ids"() -> (w1869:string[])
                      n830 = local read "Nxt T"() -> (w1863:dbl)
                      n831 = Bundle By Name(cluster=T8 {"All Param Names"=["k1"], "All Param Values"=["1.5"], "Sp IDs"=["S1", "S2", "S3"], "Sp States"=["0.000000", "0.000000", "0.000000"], "Input Equations"=["C*k1*S1", "1.5*exp(time)^(-1)"], "CompID"=["C"], "CompSize"=["3.0"], "T-Sym"="time", "T"=0.0} ("Cluster"), "All Param Names"=w1871, "All Param Values"=w1870, "Sp IDs"=w1869, "Sp States"=w1868, "Input Equations"=w1867, "CompID"=w1866, "CompSize"=w1865, "T-Sym"=w1864, "T"=w1863) -> (w1862:T8)
                      n832 = call "Value substituter in equations.vi"("Cluster"=w1862) -> ("Output Equations"=w1873:string[])
                      n833 = for {
                        tunnel: w1873 -> [w1884] mode=indexing
                        tunnel: [w1880] -> w1875 mode=indexing
                        n834 = call <vilib>:"Eval Formula String.vi"("formula"=w1884) -> ("y value"=w1881:dbl)  [unwired: 1 in, 1 out]
                        n835 = In Range and Coerce(upper limit=inf, x=w1881, lower limit=0.0) -> (coerced(x)=w1880:dbl)  [unwired: 1 out]
                      }
                      n836 = local write "Output Equations"(w1873) -> ()
                      n837 = for {
                        tunnel: w1875 -> [w1879] mode=indexing
                        shift-right: [w1878] -> w1874
                        shift-left: 0.0 -> [w1877]
                        n838 = Add(x=w1877, y=w1879) -> (x+y=w1878:dbl)
                      }
                      n839 = local write "Propensities"(w1875) -> ()
                      n840 = local write "a0"(w1874) -> ()
                    }
                    frame #7 {
                      # "next time of reaction"
                      # "next reaction value"
                      n841 = Random Number (0-1)() -> (number: 0 to 1=w1886:dbl)
                      n842 = Random Number (0-1)() -> (number: 0 to 1=w1885:dbl)
                      n843 = local write "r1"(w1886) -> ()
                      n844 = local write "r2"(w1885) -> ()
                    }
                    frame #8 {
                      # "(1/a0) * ln(1/r1)"
                      # "1/atot"
                      # "ln(1/r1)"
                      # "next reaction time"
                      n845 = local read "a0"() -> (w1892:dbl)
                      n846 = local read "r1"() -> (w1887:dbl)
                      n847 = Reciprocal(x=w1892) -> (1/x=w1889:dbl)
                      n848 = Reciprocal(x=w1887) -> (1/x=w1888:dbl)
                      n849 = Natural Logarithm(1:w1888) -> (0:w1890:dbl)
                      n850 = Compound Arithmetic op=MULTIPLY(w1889, w1890) -> (w1891:dbl)
                      n851 = local write "tau"(w1891) -> ()
                    }
                    frame #9 {
                      n852 = local read "L_cnt"() -> (w1905:i32)
                      n853 = local read "a0"() -> (w1897:dbl)
                      n854 = local read "r2"() -> (w1896:dbl)
                      n855 = local read "T"() -> (w1906:dbl[])
                      n856 = Multiply(x=w1897, y=w1896) -> (x*y=w1898:dbl)
                      n857 = local read "Continous Simulation"() -> (w1895:bool)
                      n858 = Index Array(array=w1906, index=w1905) -> (element=w1903:dbl)
                      n859 = local write "a0*r2"(w1898) -> ()
                      n860 = local read "tau"() -> (w1904:dbl)
                      n861 = Add(x=w1903, y=w1904) -> (x+y=w1894:dbl)
                      n862 = case shown="True" w1895 {
                        tunnel: w1894 -> [w1907 w1911]
                        tunnel: [w1907 w1908] -> w1893
                        frame False {
                        }
                        frame True {
                          n863 = local read "Time Limit"() -> (w1909:dbl)
                          n864 = In Range and Coerce(upper limit=w1909, x=w1911, lower limit=0.0) -> (coerced(x)=w1908:dbl)  [unwired: 1 out]
                        }
                      }
                      n865 = local read "L_cnt"() -> (w1901:i32)
                      n866 = Increment(x=w1901) -> (x+1=w1902:i32)
                      n867 = local read "T"() -> (w1900:dbl[])
                      n868 = Insert Into Array(array=w1900, index=w1902, new element=w1893) -> (w1899:dbl[])
                      n869 = local write "T"(w1899) -> ()
                    }
                    frame #10 {
                      # "Implement the selection of reaction algorithm"
                      n870 = local read "Propensities"() -> (w1913:dbl[])
                      n871 = for {
                        tunnel: w1913 -> [w1918] mode=indexing
                        shift-right: [w1916] -> _
                        shift-left: 0.0 -> [w1921]
                        i -> [w1914]
                        stop <- w1919 stop-if-true
                        n872 = local read "a0*r2"() -> (w1917:dbl)
                        n873 = Add(x=w1921, y=w1918) -> (x+y=w1916:dbl)
                        n874 = Greater?(x=w1916, y=w1917) -> (0:w1920:bool)
                        n875 = local write "Sum of Propensities for U"(w1916) -> ()
                        n876 = case shown="True" w1920 {
                          selector: w1920 -> [_ w1924]
                          tunnel: [w1922 w1924] -> w1919
                          tunnel: [w1922 w1924] -> w1915
                          tunnel: w1914 -> [_ w1923]
                          frame False {
                            w1922 = FALSE
                          }
                          frame True {
                            n877 = local write "Reac IDx"(w1923) -> ()
                          }
                        }
                        n878 = local write "Sum>a0*r2"(w1915) -> ()
                      }
                    }
                    frame #11 {
                      # "Extracting and adding the new state in the previous state of species"
                      n879 = local read "Delta Matrix"() -> (w1925:T2)
                      n880 = local read "Reac IDx"() -> (w1926:i32)
                      n881 = Index Array(array=w1925, index (row)=w1926) -> (element=w1927:T2)  [unwired: 1 in]
                      n882 = call-poly <vilib>:"Matrix To Array.vi"("Real Matrix"=w1927) -> ("Real 2D Array"=w1928:dbl[][])
                      n883 = local read "Nxt Sp State (N)"() -> (w1931:dbl[])
                      n884 = Transpose 2D Array(2D array=w1928) -> (transposed array=w1929:dbl[][])
                      n885 = Index Array(array=w1929, index (col)=0 ("disabled index (col)")) -> (element=w1932:dbl[])  [unwired: 1 in]
                      n886 = Add(x=w1932, y=w1931) -> (x+y=w1933:dbl[])
                      n887 = local write "Reac to execute"(w1932) -> ()
                      n888 = In Range and Coerce(upper limit=inf, x=w1933, lower limit=0.0) -> (coerced(x)=w1936:dbl[])  [unwired: 1 out]
                      n889 = local write "Nxt Sp State (N)"(w1936) -> ()
                    }
                  }
                  n890 = local write "All Param Values"(w1807) -> ()
                  n891 = local write "All Param Names"(w1808) -> ()
                }
              }
              "XY Graph" <- w1414
              n892 = local read "Time Limit"() -> (w1406:dbl)
              n893 = property on="XY Graph" class="XYGraph (strict)"("Smooth Update"=TRUE) -> ()  [unwired: 2 in, 2 out]
              n894 = local read "Nxt T"() -> (w1407:dbl)
              n895 = Add(x="Simulation Speed (ms)", y=u32 1 ("Simulation Speed (ms)")) -> (x+y=w1409:u32)
              n896 = Wait (ms)(milliseconds to wait=w1409) -> ()  [unwired: 1 out]
              n897 = Greater Or Equal?(x=w1407, y=w1406) -> (x >= y?=w1405:bool)
              n898 = local write "L_cnt"(w1416) -> ()
              n899 = Or(x="stop", y=w1405) -> (x .or. y?=w1403:bool)
              n900 = case shown="True" w1403 {
                selector: w1403 -> [w1417 w1421]
                tunnel: [w1417 w1421] -> w1412
                tunnel: w1411 -> [_ w1420]
                frame False {
                }
                frame True {
                  w1419 = T7."Enabled" ("Disabled")
                  n901 = property on="Threshold Value Analysis" class="Bool (strict)"("DisabledEnum"=w1419) -> ()  [unwired: 2 in, 2 out]
                  n902 = invoke on="XY Graph" class="XYGraph (strict)" method="Export Image"("FileType"=enum32{"BMP", "EPS", "EMF", "PICT"}."BMP" ("File Type"), "Target"=enum32{"File", "Clipboard"}."File", "Path"=w1420, "Overwrite"=TRUE ("Always Overwrite")) -> ()  [unwired: 4 in, 8 out]
                  n903 = property on="Simulate SBML Events" class="Bool (strict)"("DisabledEnum"=w1419) -> ()  [unwired: 2 in, 2 out]
                  n904 = property on="Modifier Degradation" class="Bool (strict)"("DisabledEnum"=w1419) -> ()  [unwired: 2 in, 2 out]
                  n905 = property on="Continous Simulation" class="Bool (strict)"("DisabledEnum"=T7."Enabled" ("Disabled")) -> ()  [unwired: 2 in, 2 out]
                }
              }
            }
            n906 = local read "DataLog"() -> (w963:path)
            n907 = stacked-sequence {
              tunnel: w963 -> [w967 _ w973]
              tunnel: w962 -> [_ _ w972]
              frame #0 {
                n908 = local read "Sp Ids"() -> (w966:string[])
                n909 = Insert Into Array(array=w966, index=0, new element="Time" ("string")) -> (w970:string[])
                n910 = call-poly <vilib>:"Write To Spreadsheet File.vi"("1D data"=w970, "file path (dialog if empty)"=w967) -> ()  [unwired: 6 in, 1 out]
              }
              frame #1 {
                n911 = Wait (ms)(milliseconds to wait=u32 3) -> ()  [unwired: 1 out]
              }
              frame #2 {
                n912 = call-poly <vilib>:"Write To Spreadsheet File.vi"("append to file? (new file:F)"=TRUE, "2D data"=w972, "file path (dialog if empty)"=w973) -> ()  [unwired: 5 in, 1 out]
              }
            }
            n913 = local read "Simulate SBML Events"() -> (w964:bool)
            n914 = case shown="True" w964 {
              frame False {
              }
              frame True {
                n915 = local read "Event Info"() -> (w985:T1)
                n916 = Unbundle By Name(w985) -> ("Delay"=w981:string[], "Priority"=w983:string[])
                n917 = Fract/Exp String To Number(string=w981) -> (number=→"Delay":dbl[])  [unwired: 3 in, 1 out]
                n918 = Fract/Exp String To Number(string=w983) -> (number=→"Priority":dbl[])  [unwired: 3 in, 1 out]
                n919 = Array Size(array=w981) -> (size(s)=w978:i32)
                n920 = Initialize Array(0 ("element"), w978) -> (→"Flag":i32[])
                n921 = Initialize Array(0.0 ("element"), w978) -> (→"Delay Val Tot":dbl[])
                n922 = while {
                  tunnel: [w989] -> _
                  i -> [w989]
                  stop <- w993 stop-if-true
                  n923 = local read "Math Val"() -> (w996:string[])
                  n924 = local read "Log Data"() -> (w998:dbl[])
                  n925 = local read "Math Op"() -> (w997:string[])
                  n926 = local read "Var Idx"() -> (w995:i32[])
                  n927 = local read "All Variables"() -> (w986:string[])
                  n928 = local read "Assign Var Idx"() -> (w987:i32[][])
                  n929 = local read "Simulation Speed (ms)"() -> (w1000:u32)
                  n930 = local read "Assign Val"() -> (w988:string[][])
                  n931 = Add(x=w1000, y=u32 1 ("Simulation Speed (ms)")) -> (x+y=w1001:u32)
                  n932 = Wait (ms)(milliseconds to wait=w1001) -> ()  [unwired: 1 out]
                  n933 = disable-structure shown="Enabled" {
                    disable-tunnel: w997 -> [w1008 _]
                    disable-tunnel: w996 -> [w1007 _]
                    disable-tunnel: w995 -> [w1006 _]
                    disable-tunnel: [w1003 _] -> _
                    disable-tunnel: w998 -> [w1005 _]
                    disable-tunnel: w988 -> [w1004 _]
                    disable-tunnel: w987 -> [w1003 _]
                    disable-tunnel: w986 -> [w1002 _]
                    frame Enabled {
                      n934 = for {
                        tunnel: w1008 -> [w1022] mode=indexing
                        tunnel: w1007 -> [w1011] mode=indexing
                        tunnel: w1006 -> [w1016] mode=indexing
                        tunnel: w1004 -> [w1019] mode=indexing
                        tunnel: w1003 -> [w1021] mode=indexing
                        tunnel: w1005 -> [w1009]
                        tunnel: w1002 -> [w1012]
                        i -> [w1020]
                        stop <- w1017 stop-if-true
                        n935 = Search 1D Array(1D array=w1012, element=w1011) -> (index of element=w1010:i32)  [unwired: 1 in]
                        n936 = Index Array(array=w1009, index=0 ("disabled index (col)")) -> (element=w1013:dbl)
                        n937 = Index Array(array=w1009, index=w1016) -> (element=w1015:dbl)
                        n938 = case shown="-1" w1010 {
                          selector: w1010 -> [w1024 _]
                          tunnel: [w1023 w1026] -> w1018
                          tunnel: w1011 -> [_ w1027]
                          tunnel: w1009 -> [w1025 _]
                          frame 0, Default {
                            n939 = Index Array(array=w1025, index=w1024) -> (element=w1023:dbl)
                          }
                          frame -1 {
                            n940 = call <vilib>:"Eval Formula String.vi"("formula"=w1027) -> ("y value"=w1026:dbl)  [unwired: 1 in, 1 out]
                          }
                        }
                        n941 = case "Math Operators" shown="\"<\"" w1022 {
                          tunnel: w1018 -> [_ w1032 w1124 w1216 w1314]
                          tunnel: w1019 -> [_ w1029 w1121 w1215 w1311]
                          tunnel: w1021 -> [_ w1028 w1120 w1214 w1310]
                          tunnel: w1015 -> [_ w1031 w1123 w1212 w1313]
                          tunnel: w1013 -> [_ w1030 w1122 w1213 w1312]
                          frame "False", Default {
                          }
                          frame "<" {
                            n942 = stacked-sequence {
                              tunnel: w1032 -> [_ w1045]
                              tunnel: w1029 -> [_ w1039]
                              tunnel: w1030 -> [_ w1038]
                              tunnel: w1031 -> [_ w1037]
                              tunnel: w1028 -> [_ w1036]
                              frame #0 {
                                # "Checking if delay is present"
                                n943 = local read "Event Idx"() -> (w1034:i32)
                                n944 = local read "Delay"() -> (w1035:dbl[])
                                n945 = Index Array(array=w1035, index=w1034) -> (element=w1033:dbl)
                                n946 = local write "Delay Val"(w1033) -> ()
                              }
                              frame #1 {
                                n947 = flat-sequence {
                                tunnel: w1037 -> [w1055]
                                tunnel: w1045 -> [w1054]
                                tunnel: w1038 -> [w1053]
                                tunnel: [w1048] -> w1044
                                tunnel: [w1047] -> w1043
                                tunnel: [w1053] -> w1042
                                tunnel: w1044 -> [w1057]
                                tunnel: w1043 -> [w1058]
                                tunnel: w1042 -> [w1056]
                                tunnel: [w1058] -> w1041
                                tunnel: [w1056] -> w1040
                                tunnel: w1041 -> [w1065]
                                tunnel: w1040 -> [w1066]
                                tunnel: w1036 -> [w1067]
                                tunnel: w1039 -> [w1068]
                                frame #0 {
                                n948 = local read "Event Idx"() -> (w1051:i32)
                                n949 = local read "Flag"() -> (w1046:i32[])
                                n950 = Less?(x=w1055, y=w1054) -> (x < y?=w1047:bool)
                                n951 = Index Array(array=w1046, index=w1051) -> (element=w1050:i32)
                                n952 = Increment(x=w1050) -> (x+1=w1049:i32)
                                n953 = Select(t=w1049, s=w1047, f=w1050) -> (s? t:f=w1048:i32)
                                n954 = Replace Array Subset(array=w1046, new element=w1048, index=w1051) -> (w1052:i32[])
                                n955 = local write "Flag"(w1052) -> ()
                                }
                                frame #1 {
                                n956 = case shown="1" w1057 {
                                tunnel: w1056 -> [_ w1063]
                                frame 0, Default {
                                }
                                frame 1 {
                                n957 = local read "Delay Val Tot"() -> (w1062:dbl[])
                                n958 = local read "Event Idx"() -> (w1060:i32)
                                n959 = local read "Delay Val"() -> (w1064:dbl)
                                n960 = Add(x=w1063, y=w1064) -> (x+y=w1059:dbl)
                                n961 = Replace Array Subset(array=w1062, new element=w1059, index=w1060) -> (w1061:dbl[])
                                n962 = local write "Delay Val Tot"(w1061) -> ()
                                }
                                }
                                }
                                frame #2 {
                                n963 = case shown="True" w1065 {
                                selector: w1065 -> [_ w1069]
                                tunnel: w1068 -> [_ w1072]
                                tunnel: w1067 -> [_ w1071]
                                tunnel: w1066 -> [_ w1070]
                                frame False {
                                }
                                frame True {
                                n964 = stacked-sequence {
                                tunnel: w1072 -> [w1076 _]
                                tunnel: w1071 -> [w1075 _]
                                tunnel: w1070 -> [w1074 _]
                                tunnel: w1069 -> [w1073 _]
                                frame #0 {
                                n965 = for {
                                tunnel: w1073 -> [w1101]
                                tunnel: w1074 -> [w1100]
                                tunnel: w1075 -> [w1080] mode=indexing
                                tunnel: w1076 -> [w1082] mode=indexing
                                n966 = local read "All Param Names"() -> (w1084:string[])
                                n967 = local read "Nxt Sp State (N)"() -> (w1081:dbl[])
                                n968 = Decrement(x=w1080) -> (x-1=w1079:i32)
                                n969 = Search 1D Array(1D array=w1084, element=w1082) -> (index of element=w1083:i32)  [unwired: 1 in]
                                n970 = case shown="0, Default" w1083 {
                                selector: w1083 -> [w1105 _]
                                tunnel: w1082 -> [_ w1107]
                                tunnel: [w1104 w1107] -> w1078
                                frame 0, Default {
                                n971 = local read "All Param Values"() -> (w1106:string[])
                                n972 = Index Array(array=w1106, index=w1105) -> (element=w1104:string)
                                }
                                frame -1 {
                                }
                                }
                                n973 = Index Array(array=w1081, index=w1079) -> (element=w1085:dbl)
                                n974 = call <vilib>:"Eval Formula String.vi"("formula"=w1078) -> ("y value"=w1077:dbl)  [unwired: 1 in, 1 out]
                                n975 = local read "Delay Val Tot"() -> (w1099:dbl[])
                                n976 = local read "Event Idx"() -> (w1098:i32)
                                n977 = Index Array(array=w1099, index=w1098) -> (element=w1097:dbl)
                                n978 = local read "All Variables"() -> (w1096:string[])
                                n979 = Greater Or Equal?(x=w1100, y=w1097) -> (x >= y?=w1102:bool)
                                n980 = And(x=w1101, y=w1102) -> (x .and. y?=w1103:bool)
                                n981 = local read "Ex_Mod_IDs"() -> (w1095:string[])
                                n982 = Select(t=w1077, s=w1103, f=w1085) -> (s? t:f=w1086:dbl)
                                n983 = Index Array(array=w1096, index=w1080) -> (element=w1089:string)
                                n984 = local read "External Modifiers"() -> (w1094:T3[])
                                n985 = Search 1D Array(1D array=w1095, element=w1089) -> (index of element=w1090:i32)  [unwired: 1 in]
                                n986 = local read "Nxt Sp State (N)"() -> (w1087:dbl[])
                                n987 = Index Array(array=w1094, index=w1090) -> (element=w1093:T3)
                                n988 = Bundle By Name(cluster=w1093, "Dial"=w1086, "String 2"=w1089) -> (w1091:T3)
                                n989 = Replace Array Subset(array=w1087, new element=w1086, index=w1079) -> (w1088:dbl[])
                                n990 = Replace Array Subset(array=w1094, new element=w1091, index=w1090) -> (w1092:T3[])
                                n991 = local write "External Modifiers"(w1092) -> ()
                                n992 = local write "Nxt Sp State (N)"(w1088) -> ()
                                }
                                }
                                frame #1 {
                                n993 = local read "Event Idx"() -> (w1115:i32)
                                n994 = local read "Event Idx"() -> (w1113:i32)
                                n995 = local read "Event Idx"() -> (w1118:i32)
                                n996 = local read "Math Val"() -> (w1114:string[])
                                n997 = local read "Var Idx"() -> (w1111:i32[])
                                n998 = local read "Math Op"() -> (w1119:string[])
                                n999 = Delete From Array(array=w1114, length=1, index=w1115) -> (array with subset deleted=w1109:string[])  [unwired: 1 out]
                                n1000 = Delete From Array(array=w1111, length=1, index=w1113) -> (array with subset deleted=w1108:i32[])  [unwired: 1 out]
                                n1001 = Delete From Array(array=w1119, length=1, index=w1118) -> (array with subset deleted=w1110:string[])  [unwired: 1 out]
                                n1002 = local write "Math Op"(w1110) -> ()
                                n1003 = local write "Math Val"(w1109) -> ()
                                n1004 = local write "Var Idx"(w1108) -> ()
                                }
                                }
                                }
                                }
                                }
                                }
                              }
                            }
                          }
                          frame ">" {
                            n1005 = stacked-sequence {
                              tunnel: w1124 -> [_ w1137]
                              tunnel: w1121 -> [_ w1131]
                              tunnel: w1122 -> [_ w1130]
                              tunnel: w1123 -> [_ w1129]
                              tunnel: w1120 -> [_ w1128]
                              frame #0 {
                                # "Checking if delay is present"
                                n1006 = local read "Event Idx"() -> (w1126:i32)
                                n1007 = local read "Delay"() -> (w1127:dbl[])
                                n1008 = Index Array(array=w1127, index=w1126) -> (element=w1125:dbl)
                                n1009 = local write "Delay Val"(w1125) -> ()
                              }
                              frame #1 {
                                n1010 = flat-sequence {
                                tunnel: w1129 -> [w1147]
                                tunnel: w1137 -> [w1146]
                                tunnel: w1130 -> [w1145]
                                tunnel: [w1140] -> w1136
                                tunnel: [w1139] -> w1135
                                tunnel: [w1145] -> w1134
                                tunnel: w1136 -> [w1149]
                                tunnel: w1135 -> [w1150]
                                tunnel: w1134 -> [w1148]
                                tunnel: [w1150] -> w1133
                                tunnel: [w1148] -> w1132
                                tunnel: w1133 -> [w1157]
                                tunnel: w1132 -> [w1158]
                                tunnel: w1128 -> [w1159]
                                tunnel: w1131 -> [w1160]
                                frame #0 {
                                n1011 = local read "Event Idx"() -> (w1143:i32)
                                n1012 = local read "Flag"() -> (w1138:i32[])
                                n1013 = Greater?(x=w1147, y=w1146) -> (0:w1139:bool)
                                n1014 = Index Array(array=w1138, index=w1143) -> (element=w1142:i32)
                                n1015 = Increment(x=w1142) -> (x+1=w1141:i32)
                                n1016 = Select(t=w1141, s=w1139, f=w1142) -> (s? t:f=w1140:i32)
                                n1017 = Replace Array Subset(array=w1138, new element=w1140, index=w1143) -> (w1144:i32[])
                                n1018 = local write "Flag"(w1144) -> ()
                                }
                                frame #1 {
                                n1019 = case shown="1" w1149 {
                                tunnel: w1148 -> [_ w1155]
                                frame 0, Default {
                                }
                                frame 1 {
                                n1020 = local read "Delay Val Tot"() -> (w1154:dbl[])
                                n1021 = local read "Event Idx"() -> (w1152:i32)
                                n1022 = local read "Delay Val"() -> (w1156:dbl)
                                n1023 = Add(x=w1155, y=w1156) -> (x+y=w1151:dbl)
                                n1024 = Replace Array Subset(array=w1154, new element=w1151, index=w1152) -> (w1153:dbl[])
                                n1025 = local write "Delay Val Tot"(w1153) -> ()
                                }
                                }
                                }
                                frame #2 {
                                n1026 = case shown="True" w1157 {
                                selector: w1157 -> [_ w1161]
                                tunnel: w1160 -> [_ w1164]
                                tunnel: w1159 -> [_ w1163]
                                tunnel: w1158 -> [_ w1162]
                                frame False {
                                }
                                frame True {
                                n1027 = stacked-sequence {
                                tunnel: w1164 -> [w1168 _]
                                tunnel: w1163 -> [w1167 _]
                                tunnel: w1162 -> [w1166 _]
                                tunnel: w1161 -> [w1165 _]
                                frame #0 {
                                n1028 = for {
                                tunnel: w1165 -> [w1193]
                                tunnel: w1166 -> [w1192]
                                tunnel: w1167 -> [w1172] mode=indexing
                                tunnel: w1168 -> [w1174] mode=indexing
                                n1029 = local read "All Param Names"() -> (w1176:string[])
                                n1030 = local read "Nxt Sp State (N)"() -> (w1173:dbl[])
                                n1031 = Decrement(x=w1172) -> (x-1=w1171:i32)
                                n1032 = Search 1D Array(1D array=w1176, element=w1174) -> (index of element=w1175:i32)  [unwired: 1 in]
                                n1033 = case shown="0, Default" w1175 {
                                selector: w1175 -> [w1197 _]
                                tunnel: w1174 -> [_ w1199]
                                tunnel: [w1196 w1199] -> w1170
                                frame 0, Default {
                                n1034 = local read "All Param Values"() -> (w1198:string[])
                                n1035 = Index Array(array=w1198, index=w1197) -> (element=w1196:string)
                                }
                                frame -1 {
                                }
                                }
                                n1036 = Index Array(array=w1173, index=w1171) -> (element=w1177:dbl)
                                n1037 = call <vilib>:"Eval Formula String.vi"("formula"=w1170) -> ("y value"=w1169:dbl)  [unwired: 1 in, 1 out]
                                n1038 = local read "Delay Val Tot"() -> (w1191:dbl[])
                                n1039 = local read "Event Idx"() -> (w1190:i32)
                                n1040 = Index Array(array=w1191, index=w1190) -> (element=w1189:dbl)
                                n1041 = local read "All Variables"() -> (w1188:string[])
                                n1042 = Greater Or Equal?(x=w1192, y=w1189) -> (x >= y?=w1194:bool)
                                n1043 = And(x=w1193, y=w1194) -> (x .and. y?=w1195:bool)
                                n1044 = local read "Ex_Mod_IDs"() -> (w1187:string[])
                                n1045 = Select(t=w1169, s=w1195, f=w1177) -> (s? t:f=w1178:dbl)
                                n1046 = Index Array(array=w1188, index=w1172) -> (element=w1181:string)
                                n1047 = local read "External Modifiers"() -> (w1186:T3[])
                                n1048 = Search 1D Array(1D array=w1187, element=w1181) -> (index of element=w1182:i32)  [unwired: 1 in]
                                n1049 = local read "Nxt Sp State (N)"() -> (w1179:dbl[])
                                n1050 = Index Array(array=w1186, index=w1182) -> (element=w1185:T3)
                                n1051 = Bundle By Name(cluster=w1185, "Dial"=w1178, "String 2"=w1181) -> (w1183:T3)
                                n1052 = Replace Array Subset(array=w1179, new element=w1178, index=w1171) -> (w1180:dbl[])
                                n1053 = Replace Array Subset(array=w1186, new element=w1183, index=w1182) -> (w1184:T3[])
                                n1054 = local write "External Modifiers"(w1184) -> ()
                                n1055 = local write "Nxt Sp State (N)"(w1180) -> ()
                                }
                                }
                                frame #1 {
                                n1056 = local read "Event Idx"() -> (w1207:i32)
                                n1057 = local read "Event Idx"() -> (w1205:i32)
                                n1058 = local read "Event Idx"() -> (w1210:i32)
                                n1059 = local read "Math Val"() -> (w1206:string[])
                                n1060 = local read "Var Idx"() -> (w1203:i32[])
                                n1061 = local read "Math Op"() -> (w1211:string[])
                                n1062 = Delete From Array(array=w1206, length=1, index=w1207) -> (array with subset deleted=w1201:string[])  [unwired: 1 out]
                                n1063 = Delete From Array(array=w1203, length=1, index=w1205) -> (array with subset deleted=w1200:i32[])  [unwired: 1 out]
                                n1064 = Delete From Array(array=w1211, length=1, index=w1210) -> (array with subset deleted=w1202:string[])  [unwired: 1 out]
                                n1065 = local write "Math Op"(w1202) -> ()
                                n1066 = local write "Math Val"(w1201) -> ()
                                n1067 = local write "Var Idx"(w1200) -> ()
                                }
                                }
                                }
                                }
                                }
                                }
                              }
                            }
                          }
                          frame ">=" {
                            n1068 = stacked-sequence {
                              tunnel: w1216 -> [_ w1229]
                              tunnel: w1215 -> [_ w1223]
                              tunnel: w1214 -> [_ w1222]
                              tunnel: w1213 -> [_ w1221]
                              tunnel: w1212 -> [_ w1220]
                              frame #0 {
                                # "Checking if delay is present"
                                n1069 = local read "Event Idx"() -> (w1218:i32)
                                n1070 = local read "Delay"() -> (w1219:dbl[])
                                n1071 = Index Array(array=w1219, index=w1218) -> (element=w1217:dbl)
                                n1072 = local write "Delay Val"(w1217) -> ()
                              }
                              frame #1 {
                                n1073 = flat-sequence {
                                tunnel: w1220 -> [w1239]
                                tunnel: w1229 -> [w1238]
                                tunnel: w1221 -> [w1237]
                                tunnel: [w1232] -> w1228
                                tunnel: [w1231] -> w1227
                                tunnel: [w1237] -> w1226
                                tunnel: w1228 -> [w1241]
                                tunnel: w1227 -> [w1242]
                                tunnel: w1226 -> [w1240]
                                tunnel: [w1242] -> w1225
                                tunnel: [w1240] -> w1224
                                tunnel: w1225 -> [w1249]
                                tunnel: w1224 -> [w1250]
                                tunnel: w1222 -> [w1251]
                                tunnel: w1223 -> [w1252]
                                frame #0 {
                                n1074 = local read "Event Idx"() -> (w1235:i32)
                                n1075 = local read "Flag"() -> (w1230:i32[])
                                n1076 = Greater Or Equal?(x=w1239, y=w1238) -> (x >= y?=w1231:bool)
                                n1077 = Index Array(array=w1230, index=w1235) -> (element=w1234:i32)
                                n1078 = Increment(x=w1234) -> (x+1=w1233:i32)
                                n1079 = Select(t=w1233, s=w1231, f=w1234) -> (s? t:f=w1232:i32)
                                n1080 = Replace Array Subset(array=w1230, new element=w1232, index=w1235) -> (w1236:i32[])
                                n1081 = local write "Flag"(w1236) -> ()
                                }
                                frame #1 {
                                n1082 = case shown="1" w1241 {
                                tunnel: w1240 -> [_ w1247]
                                frame 0, Default {
                                }
                                frame 1 {
                                n1083 = local read "Delay Val Tot"() -> (w1246:dbl[])
                                n1084 = local read "Event Idx"() -> (w1244:i32)
                                n1085 = local read "Delay Val"() -> (w1248:dbl)
                                n1086 = Add(x=w1247, y=w1248) -> (x+y=w1243:dbl)
                                n1087 = Replace Array Subset(array=w1246, new element=w1243, index=w1244) -> (w1245:dbl[])
                                n1088 = local write "Delay Val Tot"(w1245) -> ()
                                }
                                }
                                }
                                frame #2 {
                                n1089 = case shown="True" w1249 {
                                selector: w1249 -> [_ w1253]
                                tunnel: w1252 -> [_ w1256]
                                tunnel: w1251 -> [_ w1255]
                                tunnel: w1250 -> [_ w1254]
                                frame False {
                                }
                                frame True {
                                n1090 = stacked-sequence {
                                tunnel: w1256 -> [w1260 _]
                                tunnel: w1255 -> [w1259 _]
                                tunnel: w1254 -> [w1258 _]
                                tunnel: w1253 -> [w1257 _]
                                frame #0 {
                                n1091 = for {
                                tunnel: w1257 -> [w1285]
                                tunnel: w1258 -> [w1284]
                                tunnel: w1259 -> [w1264] mode=indexing
                                tunnel: w1260 -> [w1266] mode=indexing
                                n1092 = local read "All Param Names"() -> (w1268:string[])
                                n1093 = local read "Nxt Sp State (N)"() -> (w1265:dbl[])
                                n1094 = Decrement(x=w1264) -> (x-1=w1263:i32)
                                n1095 = Search 1D Array(1D array=w1268, element=w1266) -> (index of element=w1267:i32)  [unwired: 1 in]
                                n1096 = case shown="0, Default" w1267 {
                                selector: w1267 -> [w1289 _]
                                tunnel: w1266 -> [_ w1291]
                                tunnel: [w1288 w1291] -> w1262
                                frame 0, Default {
                                n1097 = local read "All Param Values"() -> (w1290:string[])
                                n1098 = Index Array(array=w1290, index=w1289) -> (element=w1288:string)
                                }
                                frame -1 {
                                }
                                }
                                n1099 = Index Array(array=w1265, index=w1263) -> (element=w1269:dbl)
                                n1100 = call <vilib>:"Eval Formula String.vi"("formula"=w1262) -> ("y value"=w1261:dbl)  [unwired: 1 in, 1 out]
                                n1101 = local read "Delay Val Tot"() -> (w1283:dbl[])
                                n1102 = local read "Event Idx"() -> (w1282:i32)
                                n1103 = Index Array(array=w1283, index=w1282) -> (element=w1281:dbl)
                                n1104 = local read "All Variables"() -> (w1280:string[])
                                n1105 = Greater Or Equal?(x=w1284, y=w1281) -> (x >= y?=w1286:bool)
                                n1106 = And(x=w1285, y=w1286) -> (x .and. y?=w1287:bool)
                                n1107 = local read "Ex_Mod_IDs"() -> (w1279:string[])
                                n1108 = Select(t=w1261, s=w1287, f=w1269) -> (s? t:f=w1270:dbl)
                                n1109 = Index Array(array=w1280, index=w1264) -> (element=w1273:string)
                                n1110 = local read "External Modifiers"() -> (w1278:T3[])
                                n1111 = Search 1D Array(1D array=w1279, element=w1273) -> (index of element=w1274:i32)  [unwired: 1 in]
                                n1112 = local read "Nxt Sp State (N)"() -> (w1271:dbl[])
                                n1113 = Index Array(array=w1278, index=w1274) -> (element=w1277:T3)
                                n1114 = Bundle By Name(cluster=w1277, "Dial"=w1270, "String 2"=w1273) -> (w1275:T3)
                                n1115 = Replace Array Subset(array=w1271, new element=w1270, index=w1263) -> (w1272:dbl[])
                                n1116 = Replace Array Subset(array=w1278, new element=w1275, index=w1274) -> (w1276:T3[])
                                n1117 = local write "External Modifiers"(w1276) -> ()
                                n1118 = local write "Nxt Sp State (N)"(w1272) -> ()
                                }
                                }
                                frame #1 {
                                n1119 = local read "Event Idx"() -> (w1305:i32)
                                n1120 = local read "Event Idx"() -> (w1303:i32)
                                n1121 = local read "Event Idx"() -> (w1308:i32)
                                n1122 = local read "Math Val"() -> (w1304:string[])
                                n1123 = local read "Assign Val"() -> (w1297:string[][])
                                n1124 = local read "Var Idx"() -> (w1301:i32[])
                                n1125 = local read "Math Op"() -> (w1309:string[])
                                n1126 = local read "Event Idx"() -> (w1296:i32)
                                n1127 = Delete From Array(array=w1304, length=1, index=w1305) -> (array with subset deleted=w1299:string[])  [unwired: 1 out]
                                n1128 = Delete From Array(array=w1301, length=1, index=w1303) -> (array with subset deleted=w1298:i32[])  [unwired: 1 out]
                                n1129 = Delete From Array(array=w1309, length=1, index=w1308) -> (array with subset deleted=w1300:string[])  [unwired: 1 out]
                                n1130 = Delete From Array(array=w1297, index (row)=w1296) -> (array with subset deleted=w1295:string[][])  [unwired: 2 in, 1 out]
                                n1131 = local write "Assign Val"(w1295) -> ()
                                n1132 = local write "Math Op"(w1300) -> ()
                                n1133 = local write "Math Val"(w1299) -> ()
                                n1134 = local write "Var Idx"(w1298) -> ()
                                n1135 = local read "Assign Var Idx"() -> (w1294:i32[][])
                                n1136 = local read "Event Idx"() -> (w1293:i32)
                                n1137 = Delete From Array(array=w1294, index (row)=w1293) -> (array with subset deleted=w1292:i32[][])  [unwired: 2 in, 1 out]
                                n1138 = local write "Assign Var Idx"(w1292) -> ()
                                }
                                }
                                }
                                }
                                }
                                }
                              }
                            }
                          }
                          frame "<=" {
                            n1139 = stacked-sequence {
                              tunnel: w1314 -> [_ w1327]
                              tunnel: w1311 -> [_ w1321]
                              tunnel: w1310 -> [_ w1320]
                              tunnel: w1312 -> [_ w1319]
                              tunnel: w1313 -> [_ w1318]
                              frame #0 {
                                # "Checking if delay is present"
                                n1140 = local read "Event Idx"() -> (w1316:i32)
                                n1141 = local read "Delay"() -> (w1317:dbl[])
                                n1142 = Index Array(array=w1317, index=w1316) -> (element=w1315:dbl)
                                n1143 = local write "Delay Val"(w1315) -> ()
                              }
                              frame #1 {
                                n1144 = flat-sequence {
                                tunnel: w1318 -> [w1337]
                                tunnel: w1327 -> [w1336]
                                tunnel: w1319 -> [w1335]
                                tunnel: [w1330] -> w1326
                                tunnel: [w1329] -> w1325
                                tunnel: [w1335] -> w1324
                                tunnel: w1326 -> [w1339]
                                tunnel: w1325 -> [w1340]
                                tunnel: w1324 -> [w1338]
                                tunnel: [w1340] -> w1323
                                tunnel: [w1338] -> w1322
                                tunnel: w1323 -> [w1347]
                                tunnel: w1322 -> [w1348]
                                tunnel: w1320 -> [w1349]
                                tunnel: w1321 -> [w1350]
                                frame #0 {
                                n1145 = local read "Event Idx"() -> (w1333:i32)
                                n1146 = local read "Flag"() -> (w1328:i32[])
                                n1147 = Less Or Equal?(x=w1337, y=w1336) -> (x <= y?=w1329:bool)
                                n1148 = Index Array(array=w1328, index=w1333) -> (element=w1332:i32)
                                n1149 = Increment(x=w1332) -> (x+1=w1331:i32)
                                n1150 = Select(t=w1331, s=w1329, f=w1332) -> (s? t:f=w1330:i32)
                                n1151 = Replace Array Subset(array=w1328, new element=w1330, index=w1333) -> (w1334:i32[])
                                n1152 = local write "Flag"(w1334) -> ()
                                }
                                frame #1 {
                                n1153 = case shown="1" w1339 {
                                tunnel: w1338 -> [_ w1345]
                                frame 0, Default {
                                }
                                frame 1 {
                                n1154 = local read "Delay Val Tot"() -> (w1344:dbl[])
                                n1155 = local read "Event Idx"() -> (w1342:i32)
                                n1156 = local read "Delay Val"() -> (w1346:dbl)
                                n1157 = Add(x=w1345, y=w1346) -> (x+y=w1341:dbl)
                                n1158 = Replace Array Subset(array=w1344, new element=w1341, index=w1342) -> (w1343:dbl[])
                                n1159 = local write "Delay Val Tot"(w1343) -> ()
                                }
                                }
                                }
                                frame #2 {
                                n1160 = case shown="True" w1347 {
                                selector: w1347 -> [_ w1351]
                                tunnel: w1350 -> [_ w1354]
                                tunnel: w1349 -> [_ w1353]
                                tunnel: w1348 -> [_ w1352]
                                frame False {
                                }
                                frame True {
                                n1161 = stacked-sequence {
                                tunnel: w1354 -> [w1358 _]
                                tunnel: w1353 -> [w1357 _]
                                tunnel: w1352 -> [w1356 _]
                                tunnel: w1351 -> [w1355 _]
                                frame #0 {
                                n1162 = for {
                                tunnel: w1355 -> [w1383]
                                tunnel: w1356 -> [w1382]
                                tunnel: w1357 -> [w1362] mode=indexing
                                tunnel: w1358 -> [w1364] mode=indexing
                                n1163 = local read "All Param Names"() -> (w1366:string[])
                                n1164 = local read "Nxt Sp State (N)"() -> (w1363:dbl[])
                                n1165 = Decrement(x=w1362) -> (x-1=w1361:i32)
                                n1166 = Search 1D Array(1D array=w1366, element=w1364) -> (index of element=w1365:i32)  [unwired: 1 in]
                                n1167 = case shown="0, Default" w1365 {
                                selector: w1365 -> [w1387 _]
                                tunnel: w1364 -> [_ w1389]
                                tunnel: [w1386 w1389] -> w1360
                                frame 0, Default {
                                n1168 = local read "All Param Values"() -> (w1388:string[])
                                n1169 = Index Array(array=w1388, index=w1387) -> (element=w1386:string)
                                }
                                frame -1 {
                                }
                                }
                                n1170 = Index Array(array=w1363, index=w1361) -> (element=w1367:dbl)
                                n1171 = call <vilib>:"Eval Formula String.vi"("formula"=w1360) -> ("y value"=w1359:dbl)  [unwired: 1 in, 1 out]
                                n1172 = local read "Delay Val Tot"() -> (w1381:dbl[])
                                n1173 = local read "Event Idx"() -> (w1380:i32)
                                n1174 = Index Array(array=w1381, index=w1380) -> (element=w1379:dbl)
                                n1175 = local read "All Variables"() -> (w1378:string[])
                                n1176 = Greater Or Equal?(x=w1382, y=w1379) -> (x >= y?=w1384:bool)
                                n1177 = And(x=w1383, y=w1384) -> (x .and. y?=w1385:bool)
                                n1178 = local read "Ex_Mod_IDs"() -> (w1377:string[])
                                n1179 = Select(t=w1359, s=w1385, f=w1367) -> (s? t:f=w1368:dbl)
                                n1180 = Index Array(array=w1378, index=w1362) -> (element=w1371:string)
                                n1181 = local read "External Modifiers"() -> (w1376:T3[])
                                n1182 = Search 1D Array(1D array=w1377, element=w1371) -> (index of element=w1372:i32)  [unwired: 1 in]
                                n1183 = local read "Nxt Sp State (N)"() -> (w1369:dbl[])
                                n1184 = Index Array(array=w1376, index=w1372) -> (element=w1375:T3)
                                n1185 = Bundle By Name(cluster=w1375, "Dial"=w1368, "String 2"=w1371) -> (w1373:T3)
                                n1186 = Replace Array Subset(array=w1369, new element=w1368, index=w1361) -> (w1370:dbl[])
                                n1187 = Replace Array Subset(array=w1376, new element=w1373, index=w1372) -> (w1374:T3[])
                                n1188 = local write "External Modifiers"(w1374) -> ()
                                n1189 = local write "Nxt Sp State (N)"(w1370) -> ()
                                }
                                }
                                frame #1 {
                                n1190 = local read "Event Idx"() -> (w1397:i32)
                                n1191 = local read "Event Idx"() -> (w1395:i32)
                                n1192 = local read "Event Idx"() -> (w1400:i32)
                                n1193 = local read "Math Val"() -> (w1396:string[])
                                n1194 = local read "Var Idx"() -> (w1393:i32[])
                                n1195 = local read "Math Op"() -> (w1401:string[])
                                n1196 = Delete From Array(array=w1396, length=1, index=w1397) -> (array with subset deleted=w1391:string[])  [unwired: 1 out]
                                n1197 = Delete From Array(array=w1393, length=1, index=w1395) -> (array with subset deleted=w1390:i32[])  [unwired: 1 out]
                                n1198 = Delete From Array(array=w1401, length=1, index=w1400) -> (array with subset deleted=w1392:string[])  [unwired: 1 out]
                                n1199 = local write "Math Op"(w1392) -> ()
                                n1200 = local write "Math Val"(w1391) -> ()
                                n1201 = local write "Var Idx"(w1390) -> ()
                                }
                                }
                                }
                                }
                                }
                                }
                              }
                            }
                          }
                        }
                        n1202 = local read "stop"() -> (w1017:bool)
                        "Event Idx" <- w1020
                      }
                    }
                    frame Disabled {
                    }
                  }
                  n1203 = local read "Math Op"() -> (w992:string[])
                  n1204 = Array Size(array=w992) -> (size(s)=w991:i32)
                  n1205 = Equal To 0?(x=w991) -> (x = 0?=w990:bool)
                  n1206 = local read "stop"() -> (w994:bool)
                  n1207 = Or(x=w990, y=w994) -> (x .or. y?=w993:bool)
                }
                "Delay Val" <- 0.0 ("element")
              }
            }
          }
        }
        n1208 = local read "Modifier Degradation"() -> (w124:bool)
        n1209 = case shown="True" w124 {
          frame False {
          }
          frame True {
            n1210 = while {
              stop <- w129 stop-if-true
              n1211 = local read "Boolean"() -> (w128:bool)
              n1212 = local read "stop"() -> (w129:bool)
              n1213 = case shown="False" w128 {
                frame False {
                  n1214 = local read "Idx of Mod in Sp IDs"() -> (w132:i32[])
                  n1215 = local read "External Modifiers"() -> (w131:T3[])
                  n1216 = for {
                    tunnel: w132 -> [w139]
                    tunnel: w131 -> [w135] mode=indexing
                    tunnel: [w134] -> w130 mode=indexing
                    i -> [w133]
                    n1217 = local read "Nxt Sp State (N)"() -> (w138:dbl[])
                    n1218 = Index Array(array=w139, index=w133) -> (element=w137:i32)
                    n1219 = Index Array(array=w138, index=w137) -> (element=w136:dbl)
                    n1220 = Bundle By Name(cluster=w135, "Dial"=w136) -> (w134:T3)
                  }
                  n1221 = local write "External Modifiers"(w130) -> ()
                }
                frame True {
                }
              }
              n1222 = local read "Simulation Speed (ms)"() -> (w126:u32)
              n1223 = Add(x=w126, y=u32 1 ("Simulation Speed (ms)")) -> (x+y=w127:u32)
              n1224 = Wait (ms)(milliseconds to wait=w127) -> ()  [unwired: 1 out]
            }
          }
        }
      }
    }
  }
  n1225 = Not(x=w6) -> (.not. x?=w5:bool)
  n1226 = local write "stop"(w5) -> ()
  n1227 = local write "Stop Main"(w5) -> ()
  n1228 = disable-structure shown="Enabled" {
    disable-tunnel: w3 -> [_ _]
    frame Enabled {
      n1229 = Current VI's Menubar() -> (w1948:refnum<k9>)
      n1230 = Delete Menu Items(9:w1948) -> (3:w1947:refnum<k9>)  [unwired: 3 in, 1 out]
      n1231 = Insert Menu Items(7:string[] ["File", "Options", "Help"], 9:w1947) -> (3:w1945:refnum<k9>)  [unwired: 4 in, 2 out]
      n1232 = Insert Menu Items(5:"File" ("menu tag"), 7:string[] ["Exit"], 9:w1945) -> (3:w1938:refnum<k9>)  [unwired: 3 in, 2 out]
      n1233 = Insert Menu Items(5:"Options" ("menu tag"), 7:string[] ["External Inputs", "Mixed Signal Waveforms"] ("item tags"), 9:w1938) -> (3:w1937:refnum<k9>)  [unwired: 3 in, 2 out]
      n1234 = Insert Menu Items(5:"Help" ("menu tag"), 7:string[] ["About this Virtual Instrument"] ("item tags"), 9:w1937) -> ()  [unwired: 3 in, 3 out]
    }
    frame Disabled {
      n1235 = local read "Log Data matrix"() -> ()  [unwired: 1 out]
    }
  }
  n1236 = control-ref of="This VI"() -> (w2:refnum<vi>)
  n1237 = while {
    tunnel: [w1953] -> w7
    tunnel: w3 -> [_]
    shift-right: [w1952] -> _
    shift-left: 220 ("Splitter Position") -> [w1951]
    tunnel: w2 -> [w1950]
    stop <- w1953 stop-if-true
    n1238 = property class="VI"(reference=w1950) -> ("Panel"=w1949:refnum<vi>)  [unwired: 1 in, 2 out]
    n1239 = Wait Until Next ms Multiple(millisecond multiple=u32 50) -> ()  [unwired: 1 out]
    n1240 = event shown="[4] \"Shut Down\": Value Change" {
      selector: _ -> [_ _ _ _ _ _]
      dyn-events: _ -> [_ _ _ _ _ _]
      timeout: _ -> [_ _ _ _ _ _]
      tunnel: [w1956 _ _ _ TRUE TRUE] -> w1953
      tunnel: [w1955 w1966 w1978 w1986 w1992 w1995] -> w1952
      tunnel: w1951 -> [w1955 w1965 w1978 w1986 w1992 w1995]
      tunnel: w1949 -> [_ w1964 w1985 _ _ _]
      event Menu Selection (User) {
        n1241 = event-data() -> ("ItemTag"=w1957:string)  [unwired: 1 in, 6 out]
        n1242 = case shown="\"False\", Default" w1957 {
          tunnel: [_ TRUE _ _ _] -> w1956
          frame "False", Default {
          }
          frame "Exit" {
            w1959 = TRUE ("stop")
            n1243 = local write "stop"(w1959) -> ()
            n1244 = local write "Stop Main"(w1959) -> ()
          }
          frame "About this Virtual Instrument" {
            n1245 = local read "Model Name"() -> (w1960:string)
            n1246 = call "About VI.vi"("Model Name"=w1960) -> ()  [unwired: 11 in]
          }
          frame "External Inputs" {
            "Trig Ext Mod Selection" <- TRUE
          }
          frame "Mixed Signal Waveforms" {
            "Trig  MSW" <- TRUE
          }
        }
      }
      event "Slider": Value Change {
        n1247 = event-data() -> ("NewVal"=w1967:bool)  [unwired: 1 in, 5 out]
        n1248 = property class="Pnl"(reference=w1964) -> ("Width"=w1963:u32)  [unwired: 1 in, 2 out]
        n1249 = case shown="False" w1967 {
          tunnel: w1963 -> [w1970 w1974]
          tunnel: [w1969 w1973] -> w1966
          tunnel: w1965 -> [w1969 _]
          frame False {
            n1250 = Subtract(x=w1970, y=w1969) -> (x-y=w1968:u32)
            n1251 = property on="Splitter 3" class="Splitter"("Position"=w1968) -> ()  [unwired: 2 in, 2 out]
          }
          frame True {
            n1252 = Subtract(x=w1974, y=u32 15) -> (x-y=w1971:u32)
            n1253 = property on="Splitter 3" class="Splitter"("Position"=w1971) -> ("Position"=w1972:i32)  [unwired: 2 in, 2 out]
            n1254 = Subtract(x=w1974, y=w1972) -> (x-y=w1973:u32)
          }
        }
      }
      event Pane Size {
        n1255 = event-data() -> ("PaneRef"=w1977:refnum<vi>)  [unwired: 1 in, 5 out]
        n1256 = property class="Pnl" props=["Height"](reference=w1985) -> ()  [unwired: 1 in, 3 out]
        n1257 = property class="Pane"(reference=w1977) -> ("Height"=w1976:u32)  [unwired: 1 in, 2 out]
        n1258 = property on="Slider" class="Bool (strict)"() -> ("Height"=w1981:u32)  [unwired: 2 in, 2 out]
        n1259 = Divide(x=w1976, y=u32 2) -> (x/y=w1983:dbl)
        n1260 = Divide(x=w1981, y=u32 2) -> (x/y=w1980:dbl)
        n1261 = Subtract(x=w1983, y=w1980) -> (x-y=w1979:dbl)
        n1262 = property on="Slider" class="Bool (strict)"("Top"=w1979) -> ()  [unwired: 2 in, 2 out]
      }
      event "Continous Simulation", "Set Time Limit": Value Change {
        n1263 = event-data() -> ()  [unwired: 1 in, 6 out]
        n1264 = case shown="True" "Continous Simulation" {
          tunnel: [inf w1990] -> w1987
          frame False {
          }
          frame True {
            n1265 = Decimal String To Number(string="Set Time Limit") -> (number=w1990:i32)  [unwired: 2 in, 1 out]
          }
        }
        "Time Limit" <- w1987
      }
      event "Shut Down": Value Change {
        n1266 = event-data() -> ()  [unwired: 1 in, 6 out]
        n1267 = stacked-sequence {
          frame #0 {
            w1994 = TRUE ("stop")
            n1268 = local write "stop"(w1994) -> ()
            n1269 = local write "Stop Main"(w1994) -> ()
          }
        }
      }
      event Panel Close {
        w1996 = TRUE ("stop")
        n1270 = event-data() -> ()  [unwired: 1 in, 4 out]
        n1271 = local write "stop"(w1996) -> ()
        n1272 = local write "Stop Main"(w1996) -> ()
      }
    }
  }
  n1273 = property class="App"() -> (error out=w10:errorcluster, "App.Kind"=w8:T10)  [unwired: 2 in, 1 out]
  n1274 = call <vilib>:"Simple Error Handler.vi"("type of dialog (OK msg:1)"=w9, "error in (no error)"=w10) -> ()  [unwired: 3 in, 5 out]
  n1275 = case shown="\"Development System\"" w8 {
    tunnel: w7 -> [_ _ _]
    frame "invalid app kind", Default {
    }
    frame "Development System" {
    }
    frame "Run Time System" {
      n1276 = control-ref of="This VI"() -> (w2000:refnum<vi>)
      n1277 = invoke class="VI" method="FP.Close"(reference=w2000) -> (reference out=w1998:refnum<vi>, error out=w1999:errorcluster)  [unwired: 2 in, 1 out]
      n1278 = Close Reference(reference=w1998, error in (no error)=w1999) -> ()  [unwired: 1 out]
    }
  }
